vi "USO_GUI.vi"() -> ()   [LabVIEW 2014]
uses:
  gfitsio/cfitsio-bitpix.ctl
  <vilib>/Instr/_visa.llb/VISA Configure Serial Port (Instr).vi
  gfitsio/gfitsio.lvlib
  <vilib>/gmath/NI_Gmath.lvlib
panel:
  out "Start time Array":timestamp[](array[timestamp])
  out "End time Array":timestamp[](array[timestamp])
  in  "Voltage-Retardance file path for lcvr2":path
  in  "Start observation session":bool
  out "LCVR closing\nvariable":T1(array[cluster])
  out "LCVR variable":T2
  out "Current Lcvr Temp":dbl
  out "volt set of lcvr 2":dbl[](array[numeric]) format="%_6g"
  out "volt set of lcvr 1":dbl[](array[numeric]) format="%_6g"
  in  "Voltage-Retardance file path for lcvr1":path
  in  "LCVR Set Temperature":dbl=21.0 min=10.0 max=50.0
  out "Buf no 2":bool
  out "Buf no 1":bool
  out "hout":u64
  in  "OpenStructureIn":T3={"Size"=88, "InterfaceType"=1, "Camera Number"=0, "CameraNumAtInterface"=0, "OpenFlags"=[], "OpenDWFlags"=[], "OpenPtrs"=[]} {"InterfaceType" items=["IEEE1394/FireWire", "IEEE1394/FireWire", "Matrox Helios CameraLink", "SiliconSoftware MicroEnableIII CL", "National Instruments CameraLink", "Gigabit Ethernet", "USB", "SiliconSoftware MicroEnable IV CL", "Reserved", "Reserved", "Generic CameraLink with CLSER.DLL"]}
  out "Buff_no 2":i16
  out "Buff_no1":i16
  in  "Close USO software":bool
  in  "spectroscopy/spectropolarimetry tab":enum32{"Spectroscopy", "Spectropolarimetry"}(tab) caption="Tab Control"
  in  "Slide":cluster{i32, i32}(slide)={16384, 0} scale=0.0..16400.0
  in  "Display Intensity control":bool
  in  "Control Pannel":T4
  in  "Cam Exp (msec)":dbl
  out "Cam Delay (msec)":dbl
  in  "Scan distance (1=10nm)":dbl min=-6000.0 max=6000.0 step=0.01
  in  "Scan steps":dbl=190.0
  out "Steps performed":i32(slide) max=190 scale=0.0..190.0
  in  "Start Spectroscopy":bool
  in  "Stop Spectroscopy":bool
  out "CCD Display":i32[][](graph)
  out "Data is stored in the folder.........":path
  in  "accept intensity":bool
  in  "Averaging \nNum":dbl=1.0
  in  "Image averaging":enum32{"Per scan", "Per Polarisation"}(radio)
  in  "LCVR Temperature in deg C\n      Set         Current":dbl[](array[numeric]) min=0.0 max=50.0
  in  "Slide sp":cluster{i32, i32}(slide)={16384, 0} scale=0.0..16400.0
  in  "accept intensity sp":bool
  out "Data is stored in the folder sp.........":path
  out "CCD Display sp":i32[][](graph)
  in  "Stop Spectroscopy sp":bool
  in  "Start Spectroscopy sp":bool
  out "Steps performed sp":i32(slide) max=190 scale=0.0..10.0
  in  "Scan steps sp":dbl=190.0
  in  "Scan distance (1=10nm) sp":dbl min=-6000.0 max=6000.0 step=0.01
  out "Cam Delay (msec) sp":dbl
  in  "Cam Exp (msec) sp":dbl
  in  "Display Intensity control sp":bool
  in  "Control Pannel sp":T4
  out "Motor Variable":T5
  out "Cam Variable":T6
  in  "Move step size(1=10nm)":i32=100
  in  "VISA Refnum in":refnum<visa-resource-name>
  in  "DELAY (ms) in":u32=50
  in  "CONTROLLER Number":string="1"
  out "Status":string
  in  "Apply":bool
  in  "InterfaceType":u32(ring)=6 items=["Ethernet"=5, "USB"=6]
  in  "Finish":bool
  out "Cam Detail":T7
  in  "Delay in msec":u32 max=4233600000
  in  "Exposure in msec":u32=30 min=500 max=4233600000
  in  "Initialise Device":u16(ring)=3 items=["Camera", "Liquid crystal", "Scan mirror", "--FF--"]
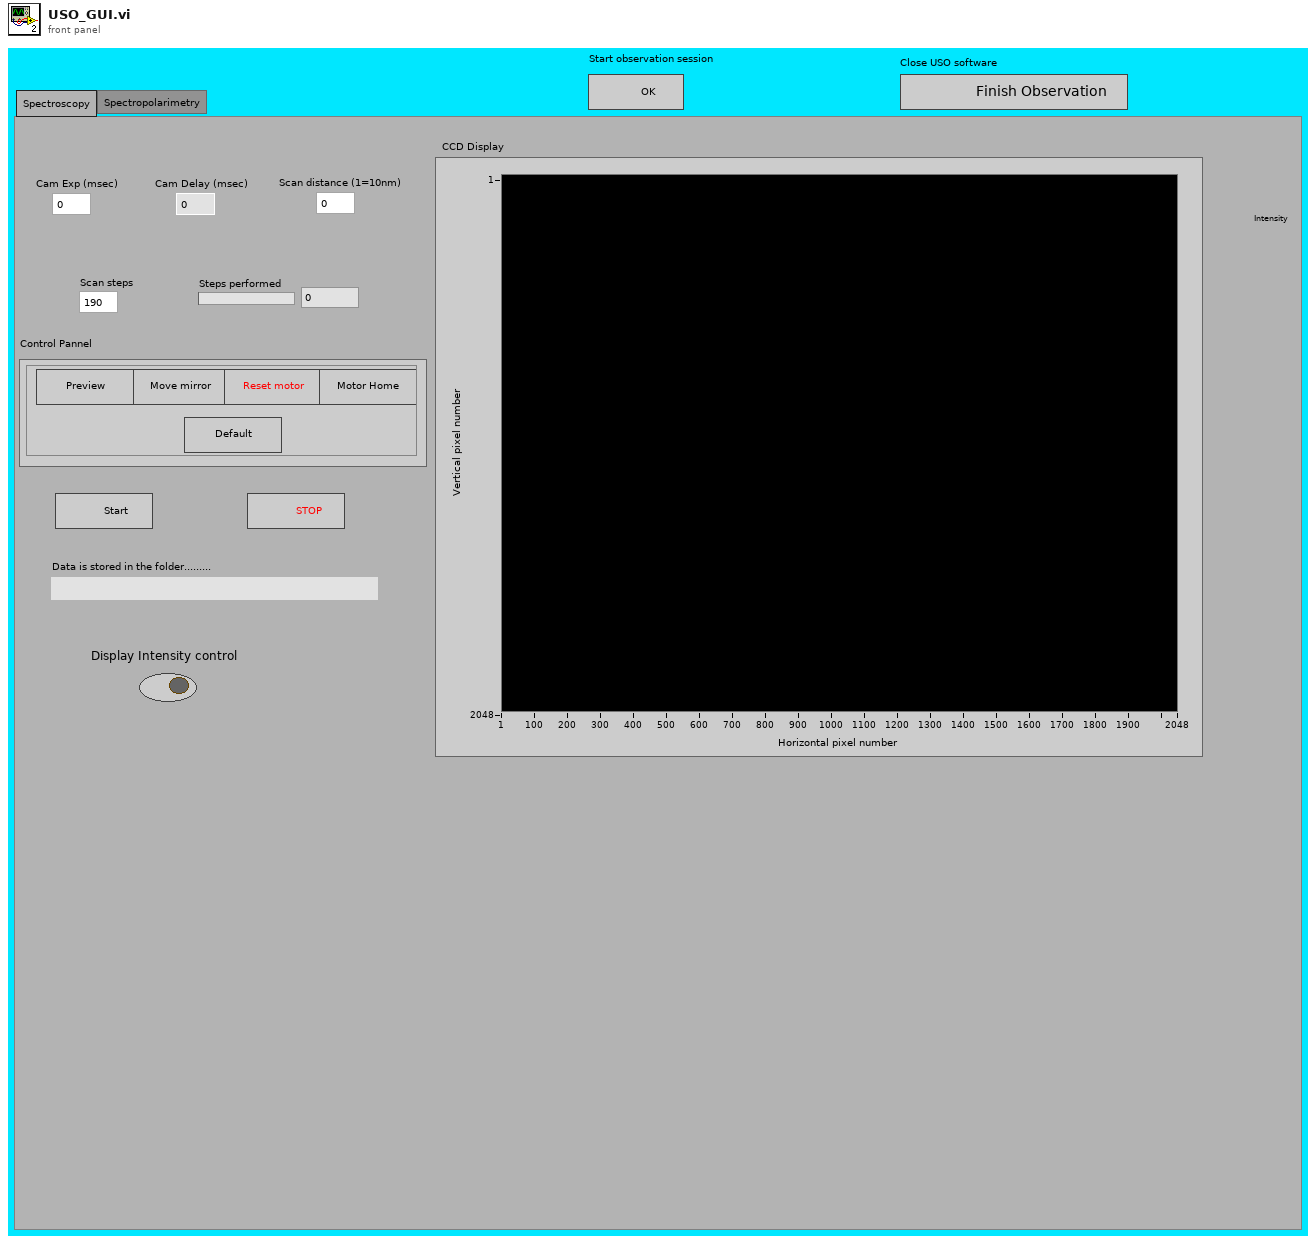
[diagram p1: front panel]
types:
  T1 = cluster{"Device Handle":u32, "Pipe 0 Handle":u32, "Pipe 1 Handle":u32}[]
  T2 = cluster{"Open USB I/O Stuff":cluster{"Device Handle":u32, "Pipe 0 Handle":u32, "Pipe 1 Handle":u32}, "volt set of lcvr 1":dbl[], "volt set of lcvr 2":dbl[], "LCVR Set Temperature":dbl, "Current Lcvr Temp":dbl}
  T3 = cluster{"Size":u16, "InterfaceType":u16, "Camera Number":u16, "CameraNumAtInterface":u16, "OpenFlags":u16[], "OpenDWFlags":u32[], "OpenPtrs":u32[]}
  T4 = cluster{"Move mirror":bool, "Preview":bool, "reset motor":bool, "motor home":bool, "Restore default values":bool}
  T5 = cluster{"Dup Controller #":string, "VISA Refnum out":refnum<visa-resource-name>, "DELAY (ms) out":u32, "Move step size":i32, "error out":errorcluster}
  T6 = cluster{"hout":u64, "ErrorOut":errorcluster, "Description":cluster{"Size":u16, "SensorTypeDESC":u16, "SensorSubtypeDESC":u16, "MaxHorizontalResStdDESC":u16, "MaxVerticalResStdDESC":u16, "MaxHorizontalResExtDESC":u16, "MaxVerticalResExtDESC":u16, "DynResDESC":u16, "MaxBinHorzDESC":u16, "BinHorzStepDESC":bool, "MaxBinVertDESC":u16, "BinVertStepDESC":bool, "ROIHorzStepDESC":u16, "ROIVertStepDESC":u16, "NumADCDESC":u16, "IRDESC":bool, "MinDelayDESC":u32, "MaxDelayDESC":u32, "MinDelayStepDESC":u32, "MinExpoDESC":u32, "MaxExpoDESC":u32, "MinExpoStepDESC":u32, "MinDelayIRDESC":u32, "MaxDelayIRDESC":u32, "MinExpoIRDESC":u32, "MaxExpoIRDESC":u32, "TimeTableDESC":bool, "DoubleImageDESC":bool, "MinCoolSetDESC":i16, "MaxCoolSetDESC":i16, "MDefaultCoolSetDESC":i16, "PowerDownModeDESC":bool, "OffsetRegDESC":bool, "ColorPattern":cluster{"UpperLeftColor":u8, "UpperRightColor":u8, "LowerLeftColor":u8, "LowerRightColor":u8}, "PatternTypeDESC":bool, "PixelRates":u32[], "CoversionFactors":u16[], "Reserved":u32[], "NoiseFilterCapable":bool, "HotPixelCapable":bool, "HotPixelWithNoiseFilter":bool, "ASCIITimeCapable":bool, "Extended Description":bool, "Get Extended":bool, "Reserved Flag 1":bool, "Reserved Flag 2":bool}}
  T7 = cluster{"Size":u16, "SensorTypeDESC":u16, "SensorSubtypeDESC":u16, "MaxHorizontalResStdDESC":u16, "MaxVerticalResStdDESC":u16, "MaxHorizontalResExtDESC":u16, "MaxVerticalResExtDESC":u16, "DynResDESC":u16, "MaxBinHorzDESC":u16, "BinHorzStepDESC":bool, "MaxBinVertDESC":u16, "BinVertStepDESC":bool, "ROIHorzStepDESC":u16, "ROIVertStepDESC":u16, "NumADCDESC":u16, "IRDESC":bool, "MinDelayDESC":u32, "MaxDelayDESC":u32, "MinDelayStepDESC":u32, "MinExpoDESC":u32, "MaxExpoDESC":u32, "MinExpoStepDESC":u32, "MinDelayIRDESC":u32, "MaxDelayIRDESC":u32, "MinExpoIRDESC":u32, "MaxExpoIRDESC":u32, "TimeTableDESC":bool, "DoubleImageDESC":bool, "MinCoolSetDESC":i16, "MaxCoolSetDESC":i16, "MDefaultCoolSetDESC":i16, "PowerDownModeDESC":bool, "OffsetRegDESC":bool, "ColorPattern":cluster{"UpperLeftColor":u8, "UpperRightColor":u8, "LowerLeftColor":u8, "LowerRightColor":u8}, "PatternTypeDESC":bool, "PixelRates":u32[], "CoversionFactors":u16[], "Reserved":u32[], "NoiseFilterCapable":bool, "HotPixelCapable":bool, "HotPixelWithNoiseFilter":bool, "ASCIITimeCapable":bool, "Extended Description":bool, "Get Extended":bool, "Reserved Flag 1":bool, "Reserved Flag 2":bool}
  T8 = enum8{"Enabled", "Disabled", "Disabled and Grayed Out"}
  T9 = enum16{"open", "open or create", "create or replace", "create", "open (read only)"}
  T10 = cluster{"Device Handle":u32, "Pipe 0 Handle":u32, "Pipe 1 Handle":u32}
  T11 = cluster{"Open USB I/O Stuff":cluster{"Device Handle":u32, "Pipe 0 Handle":u32, "Pipe 1 Handle":u32}, "yi":dbl[], "yi":dbl[], dbl, "Temp":dbl}
  T12 = cluster{"Dup Controller #":string, "VISA Refnum out":refnum<visa-resource-name>, "DELAY (ms) out":u32, "Move step size(1=10nm)":i32, "error out":errorcluster}
  T13 = cluster{"hout":u64, "error out":errorcluster, "Description":cluster{"Size":u16, "SensorTypeDESC":u16, "SensorSubtypeDESC":u16, "MaxHorizontalResStdDESC":u16, "MaxVerticalResStdDESC":u16, "MaxHorizontalResExtDESC":u16, "MaxVerticalResExtDESC":u16, "DynResDESC":u16, "MaxBinHorzDESC":u16, "BinHorzStepDESC":bool, "MaxBinVertDESC":u16, "BinVertStepDESC":bool, "ROIHorzStepDESC":u16, "ROIVertStepDESC":u16, "NumADCDESC":u16, "IRDESC":bool, "MinDelayDESC":u32, "MaxDelayDESC":u32, "MinDelayStepDESC":u32, "MinExpoDESC":u32, "MaxExpoDESC":u32, "MinExpoStepDESC":u32, "MinDelayIRDESC":u32, "MaxDelayIRDESC":u32, "MinExpoIRDESC":u32, "MaxExpoIRDESC":u32, "TimeTableDESC":bool, "DoubleImageDESC":bool, "MinCoolSetDESC":i16, "MaxCoolSetDESC":i16, "MDefaultCoolSetDESC":i16, "PowerDownModeDESC":bool, "OffsetRegDESC":bool, "ColorPattern":cluster{"UpperLeftColor":u8, "UpperRightColor":u8, "LowerLeftColor":u8, "LowerRightColor":u8}, "PatternTypeDESC":bool, "PixelRates":u32[], "CoversionFactors":u16[], "Reserved":u32[], "NoiseFilterCapable":bool, "HotPixelCapable":bool, "HotPixelWithNoiseFilter":bool, "ASCIITimeCapable":bool, "Extended Description":bool, "Get Extended":bool, "Reserved Flag 1":bool, "Reserved Flag 2":bool}}
  T14 = cluster{"Dup Controller # out":string, "VISA Refnum out":refnum<visa-resource-name>, "DELAY (ms) out":u32, "Move step size":i32, "error out":errorcluster}
  T15 = cluster{"Dup Controller #":string, "VISA Refnum out":refnum<visa-resource-name>, "Delay (ms) out ":u32, "Move step size":i32, "error out":errorcluster}
  T16 = cluster{"Dup Controller #":string, "Dup. VISA handle":refnum<visa-resource-name>, "DELAY (ms) out":u32, "Move step size":i32, "error out":errorcluster}
  T17 = typedef "gfitsio.lvlib/cfitsio-bitpix.ctl" = i32
  T18 = typedef "gfitsio.lvlib/gfitsio-refnum.ctl" = refnum<k1>
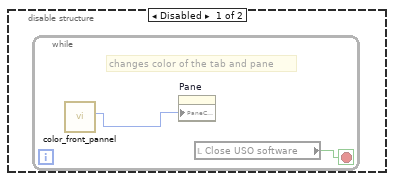
[diagram p2: hidden frame]
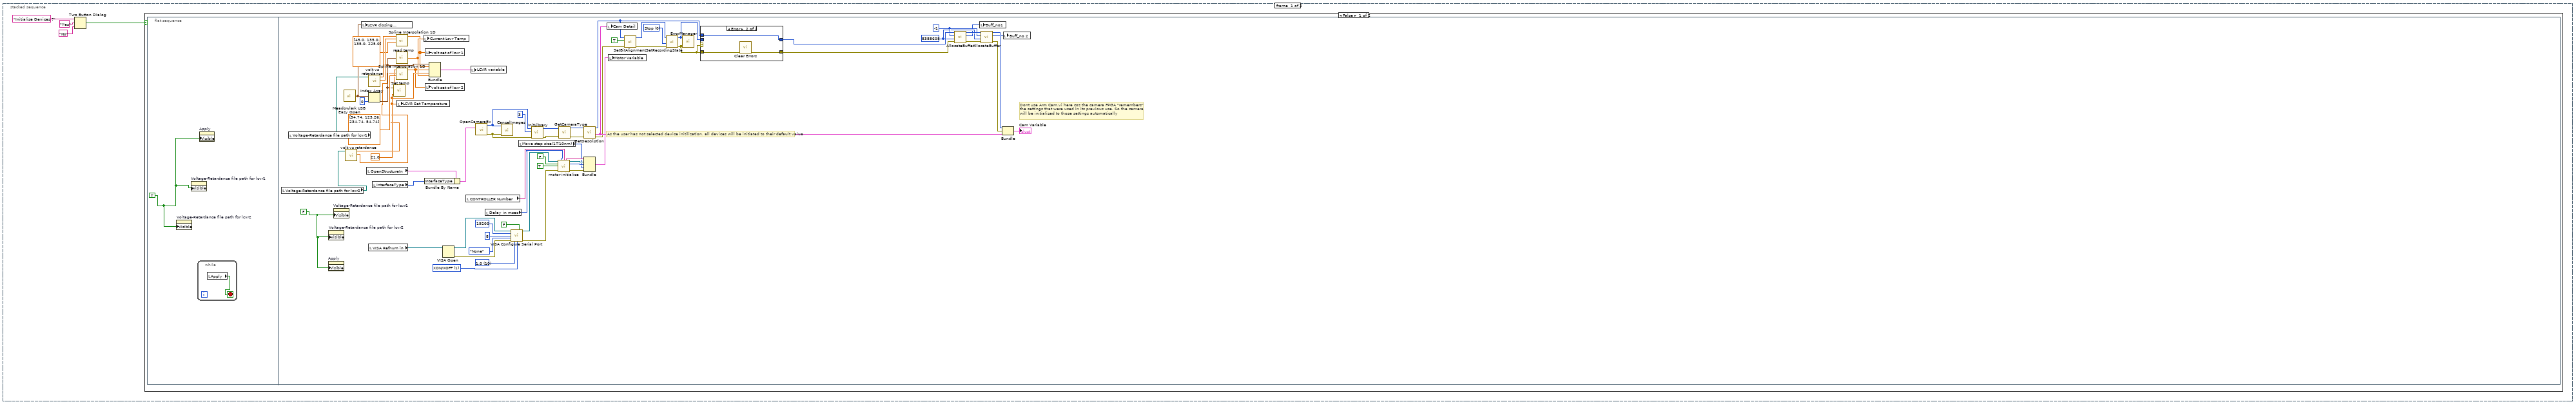
[diagram p3: hidden frame]
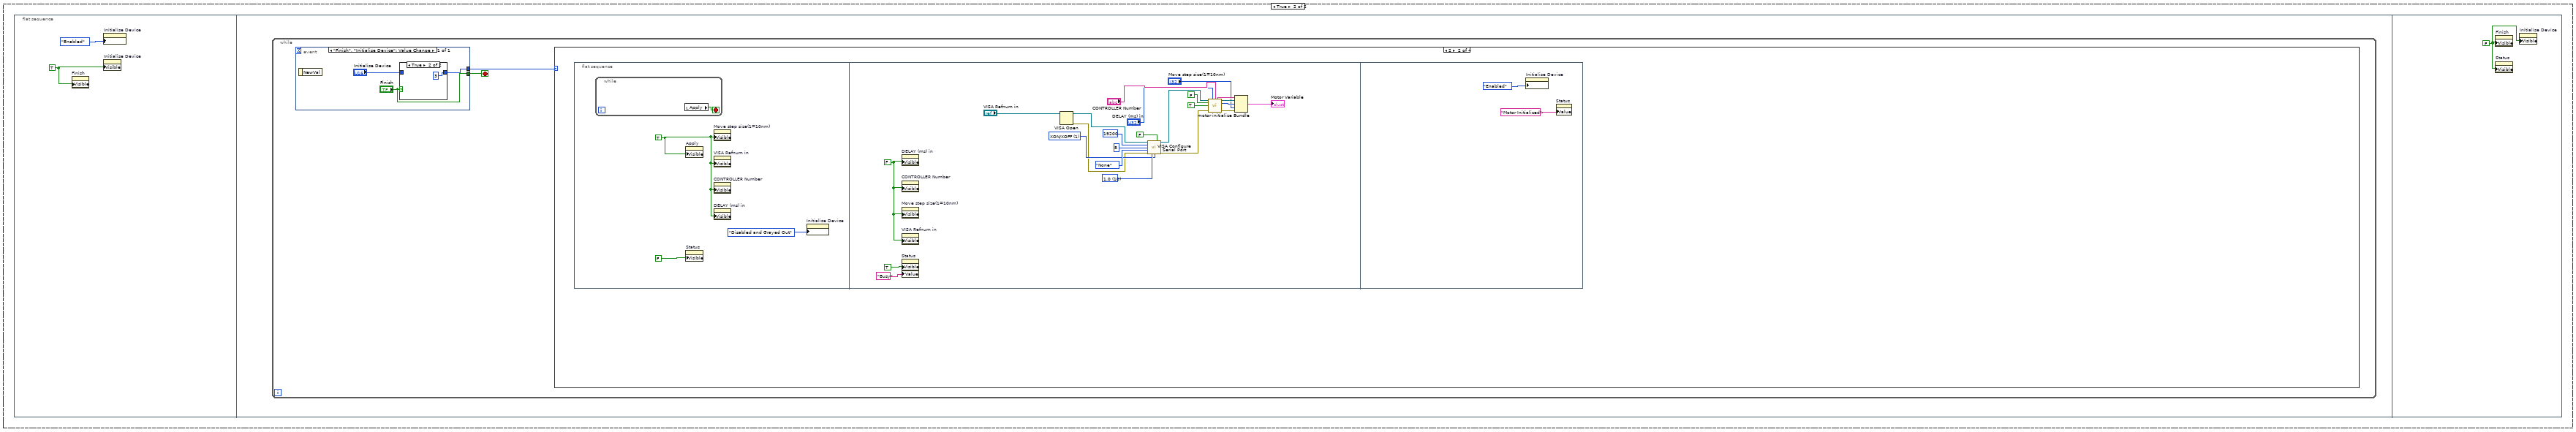
[diagram p5: hidden frame]
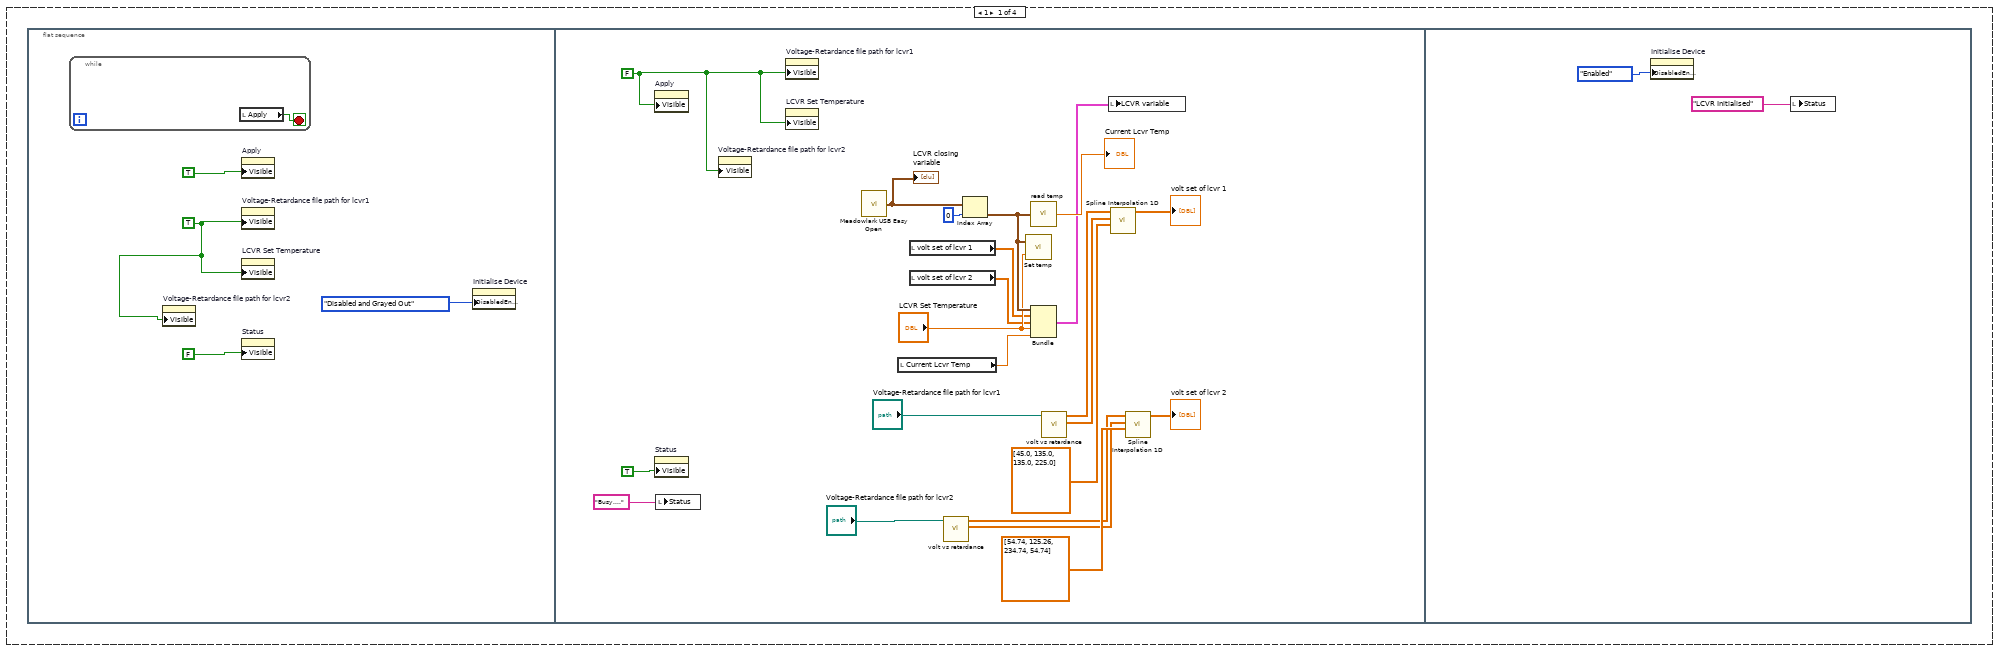
[diagram p7: hidden frame]
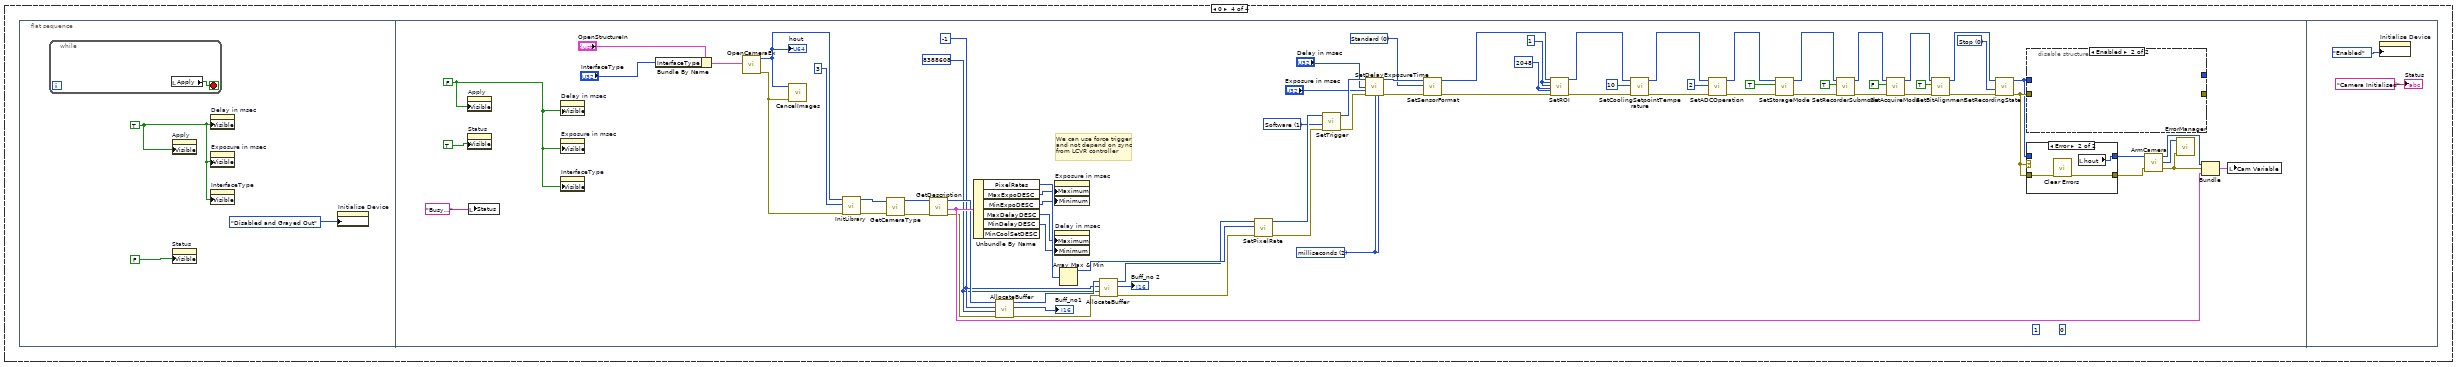
[diagram p9: hidden frame]
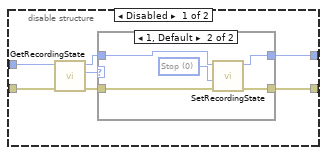
[diagram p10: hidden frame]
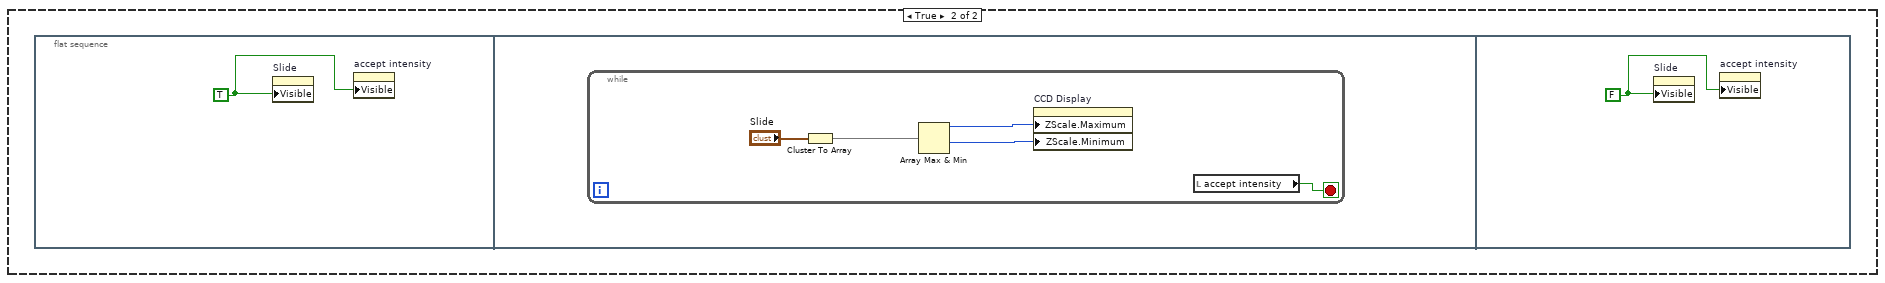
[diagram p16: hidden frame]
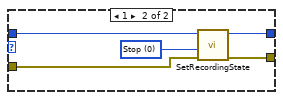
[diagram p17: hidden frame]
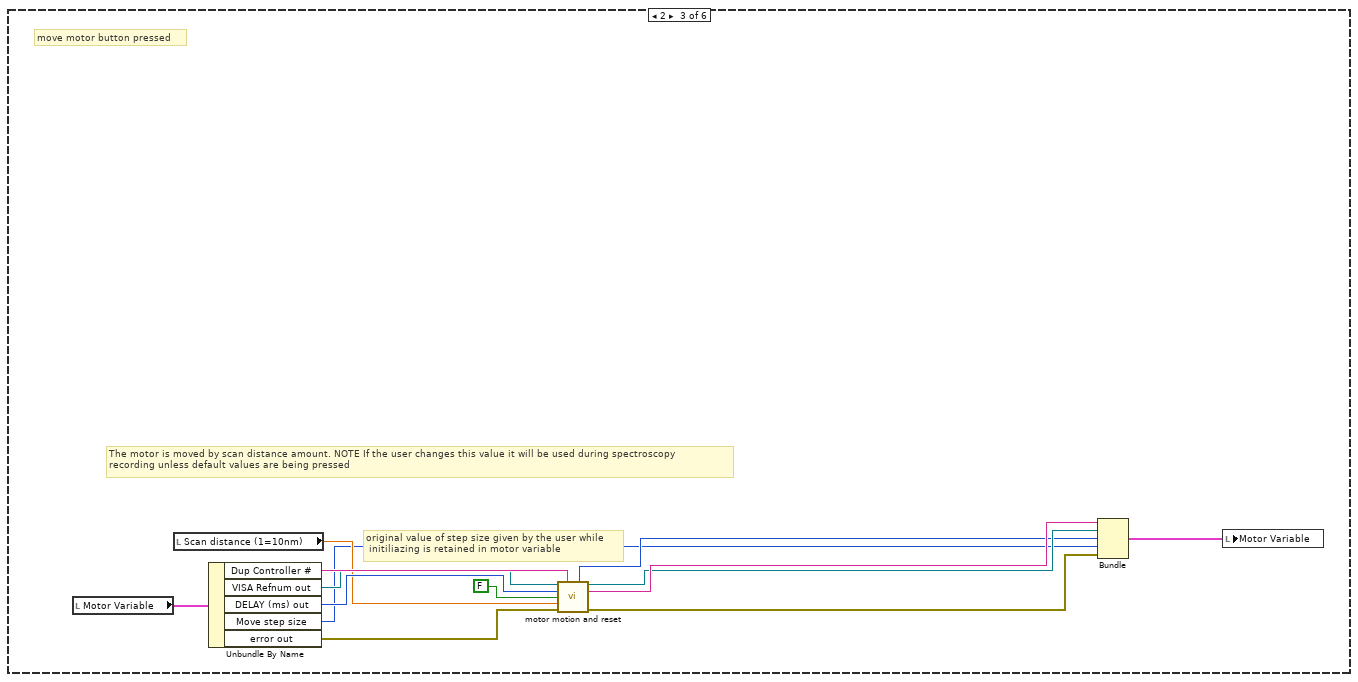
[diagram p19: hidden frame]
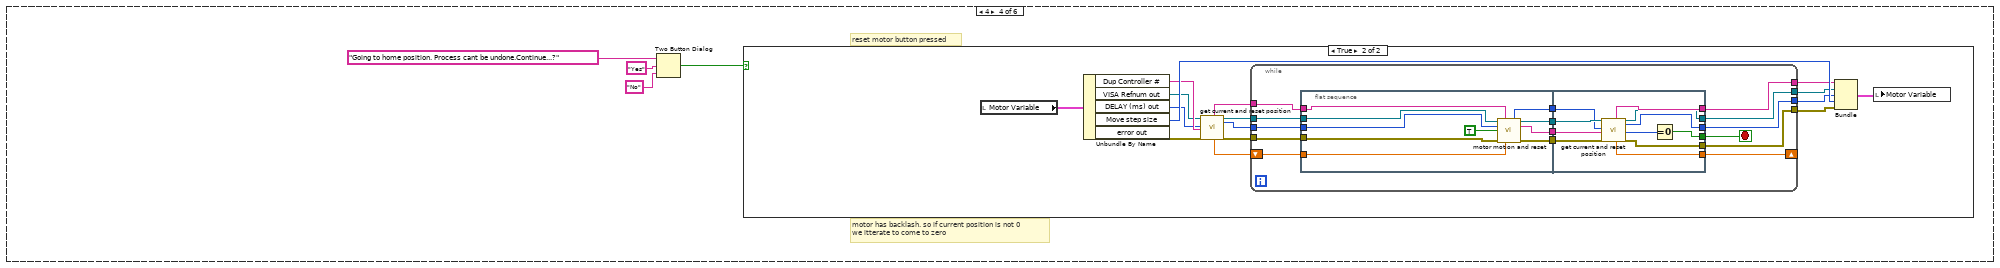
[diagram p20: hidden frame]
diagram:
  w2 = TRUE
  w3 = 2048.0 ("X Scale.Range:Maximum")
  w4 = 1.0 ("X Scale.Range:Minimum")
  w1 = FALSE
  n1 = disable-structure shown="Enabled" {
    frame Disabled {
      n2 = while {
        stop <- w6 stop-if-true
        # "changes color of the tab and pane"
        n3 = call "color_front_pannel.vi"() -> ("Resolved Color"=w5:u32)  [unwired: 11 in]
        n4 = property on="Pane" class="Pane"("PaneColor"=w5) -> ()  [unwired: 2 in, 2 out]
        n5 = local read "Close USO software"() -> (w6:bool)
      }
    }
    frame Enabled {
    }
  }
  n6 = stacked-sequence {
    frame #0 {
      n7 = Two Button Dialog(message="Initialise Devices ?", 1:"No" ("F button name (\"Cancel\")"), 2:"Yes" ("T button name (\"OK\")")) -> (T button?=w7:bool)
      n8 = case shown="False" w7 {
        frame False {
          n9 = flat-sequence {
            frame #0 {
              w11 = TRUE
              n10 = property on="Voltage-Retardance file path for lcvr2" class="Path"("Visible"=w11) -> ()  [unwired: 2 in, 2 out]
              n11 = property on="Voltage-Retardance file path for lcvr1" class="Path"("Visible"=w11) -> ()  [unwired: 2 in, 2 out]
              n12 = while {
                stop <- w12 stop-if-true
                n13 = local read "Apply"() -> (w12:bool)
              }
              n14 = property on="Apply" class="Bool (strict)"("Visible"=w11) -> ()  [unwired: 2 in, 2 out]
            }
            frame #1 {
              w13 = FALSE
              w24 = u16 1 items=["None", "XON/XOFF", "RTS/CTS", "XON/XOFF & RTS/CTS", "DTR/DSR", "XON/XOFF & DTR/DSR"] ("flow control (0:none)")
              w25 = u16 10 items=["1.0"=10, "1.5"=15, "2.0"=20] ("stop bits (10: 1 bit)")
              w39 = 21.0
              w56 = u32 8388608 ("Size")
              w57 = i16 -1 ("BufNr")
              w64 = u16 0 items=["Stop", "Run"] ("RecordingState")
              # "Dont use Arm Cam.vi here coz the camera FPGA \"remembers\"\nthe settings that were used in its previous use. So the camera \nwill be initialized to those settings automatically"
              # "As the user has not selected device initilization, all devices will be initiated to their default value"
              n15 = local read "Voltage-Retardance file path for lcvr2"() -> (w14:path)
              n16 = local read "Voltage-Retardance file path for lcvr1"() -> (w15:path)
              n17 = property on="Apply" class="Bool (strict)"("Visible"=w13) -> ()  [unwired: 2 in, 2 out]
              n18 = property on="Voltage-Retardance file path for lcvr2" class="Path"("Visible"=w13) -> ()  [unwired: 2 in, 2 out]
              n19 = property on="Voltage-Retardance file path for lcvr1" class="Path"("Visible"=w13) -> ()  [unwired: 2 in, 2 out]
              n20 = call "Meadowlark USB Easy Open.vi"() -> ("USB Device and Pipes Array"=w34:T1)  [unwired: 2 out]
              n21 = call "volt vs retardance.vi"("file path (dialog if empty)"=w14) -> ("retardance in degree(known)"=w16:dbl[], "Voltage(unknown)"=w17:dbl[])  [unwired: 9 in]
              n22 = local write "LCVR closing\nvariable"(w34) -> ()
              n23 = local read "OpenStructureIn"() -> (w51:T3)
              n24 = call "volt vs retardance.vi"("file path (dialog if empty)"=w15) -> ("retardance in degree(known)"=w44:dbl[], "Voltage(unknown)"=w43:dbl[])  [unwired: 9 in]
              n25 = Index Array(array=w34, index=0) -> (element=w40:T10)
              n26 = local read "VISA Refnum in"() -> (w20:refnum<visa-resource-name>)
              n27 = local read "InterfaceType"() -> (w49:u32)
              n28 = call "Set temp.vi"("Temp"=w39, "USB Open Device Cluster"=w40) -> ()  [unwired: 1 in]
              n29 = call <vilib>:"Spline Interpolation 1D.vi"("xi"=dbl[] [45.0, 135.0, 135.0, 225.0], "X"=w44, "Y"=w43) -> ("yi"=w37:dbl[])  [unwired: 6 in, 2 out]
              n30 = call "read temp.vi"("USB Open Device Cluster"=w40) -> ("Temp"=w38:dbl)
              n31 = call <vilib>:"Spline Interpolation 1D.vi"("xi"=dbl[] [54.74, 125.26, 234.74, 54.74], "X"=w16, "Y"=w17) -> ("yi"=w36:dbl[])  [unwired: 6 in, 2 out]
              n32 = local write "LCVR Set Temperature"(w39) -> ()
              n33 = local write "Current Lcvr Temp"(w38) -> ()
              n34 = Bundle By Name(cluster=w51, "InterfaceType"=w49) -> (w48:T3)
              n35 = local write "volt set of lcvr 1"(w37) -> ()
              n36 = local write "volt set of lcvr 2"(w36) -> ()
              n37 = Bundle("Open USB I/O Stuff"=w40, "yi"=w37, "yi"=w36, w39, "Temp"=w38) -> (w35:T11)  [unwired: 1 in]
              n38 = VISA Open(VISA resource name=w20) -> (VISA resource name=w22:refnum<visa-resource-name>, error out=w21:errorcluster)  [unwired: 4 in]
              n39 = local read "CONTROLLER Number"() -> (w71:string)
              n40 = local write "LCVR variable"(w35) -> ()
              n41 = call <userlib>:"OpenCameraEx.vi"("OpenStructureIn"=w48) -> ("error out"=w46:errorcluster, "hout"=w47:u64)  [unwired: 3 in, 2 out]
              n42 = local read "Delay in msec"() -> (w72:u32)
              n43 = call <userlib>:"CancelImages.vi"("error in (no error)"=w46, "ph"=w47) -> ()  [unwired: 1 in, 3 out]
              n44 = call-poly "VISA Configure Serial Port"("VISA resource name"=w22, "Enable Termination\nChar (T)"=FALSE ("Enable Termination\nChar (T)"), "baud rate (9600)"=u32 19200, "data bits (8)"=u16 8, "parity (0:none)"=enum16{"None", "Odd", "Even", "Mark", "Space"}."None", "error in (no error)"=w21, "stop bits (10: 1 bit)"=w25, "flow control (0:none)"=w24) -> ("VISA resource name out"=w19:refnum<visa-resource-name>, "error out"=w18:errorcluster)  [unwired: 6 in]
              n45 = local read "Move step size(1=10nm)"() -> (w66:i32)
              n46 = call <userlib>:"InitLibrary.vi"("error in (no error)"=w46, "InterfaceType"=u32 3, "ph"=w47) -> ("error out"=w79:errorcluster, "hout"=w80:u64)  [unwired: 7 in]
              n47 = call "motor initialize.vi"("VISA Refnum in"=w19, "DELAY (ms) in"=w72, "CONTROLLER"=w71, "MODE"=FALSE, "MOTOR OFF/ON"=TRUE, "error in (no error)"=w18) -> ("Dup Controller #"=w70:string, "VISA Refnum out"=w68:refnum<visa-resource-name>, "DELAY (ms) out"=w67:u32, "error out"=w65:errorcluster)  [unwired: 2 in, 4 out]
              n48 = call <userlib>:"GetCameraType.vi"("ph"=w80, "error in (no error)"=w79) -> ("hout"=w78:u64, "error out"=w77:errorcluster)  [unwired: 1 in, 2 out]
              n49 = call <userlib>:"GetDescription.vi"("ErrorIn"=w77, "ph"=w78) -> ("ErrorOut"=w30:errorcluster, "Description"=w76:T7, "hout"=w32:u64)  [unwired: 2 in, 1 out]
              n50 = Bundle("Dup Controller #"=w70, "VISA Refnum out"=w68, "DELAY (ms) out"=w67, "Move step size(1=10nm)"=w66, "error out"=w65) -> (w69:T12)  [unwired: 1 in]
              n51 = local write "Cam Detail"(w76) -> ()
              n52 = local write "Motor Variable"(w69) -> ()
              n53 = call <userlib>:"SetBitAlignment.vi"("error in (no error)"=w30, "BitAlignent"=TRUE, "ph"=w32) -> ("error out"=w29:errorcluster, "hout"=w31:u64)  [unwired: 2 in, 1 out]
              n54 = call <userlib>:"SetRecordingState.vi"("ErrorIn"=w29, "RecordingState"=w64, "ph"=w31) -> ("ErrorOut"=w52:errorcluster, "hout"=w53:u64)  [unwired: 2 in, 1 out]
              n55 = call <userlib>:"ErrorManager.vi"("ErrorIn"=w52, "ErrorCode"=w53) -> ()  [unwired: 3 in, 1 out]
              n56 = case shown="Error" w52 {
                tunnel: [w82 w84] -> w60
                tunnel: w52 -> [w82 w85]
                tunnel: w53 -> [w81 _]
                tunnel: [w81 w83] -> w63
                tunnel: w32 -> [_ w83]
                frame No Error {
                }
                frame Error {
                  n57 = call <vilib>:"Clear Errors.vi"("error in (no error)"=w85) -> ("error out"=w84:errorcluster)  [unwired: 5 in, 1 out]
                }
              }
              n58 = call <userlib>:"AllocateBuffer.vi"("error in (no error)"=w60, "Size"=w56, "BufNr"=w57, "ph"=w63) -> ("error out"=w59:errorcluster, "BufNrOut"=w55:i16, "hout"=w62:u64)  [unwired: 2 in, 3 out]
              n59 = local write "Buff_no1"(w55) -> ()
              n60 = call <userlib>:"AllocateBuffer.vi"("error in (no error)"=w59, "Size"=w56, "BufNr"=w57, "ph"=w62) -> ("error out"=w58:errorcluster, "BufNrOut"=w54:i16, "hout"=w61:u64)  [unwired: 2 in, 3 out]
              n61 = Bundle("hout"=w61, "error out"=w58, "Description"=w76) -> (→"Cam Variable":T13)  [unwired: 1 in]
              n62 = local write "Buff_no 2"(w54) -> ()
            }
          }
        }
        frame True {
          n63 = flat-sequence {
            frame #0 {
              w87 = TRUE
              n64 = property on="Finish" class="Bool"("Visible"=w87) -> ()  [unwired: 2 in, 2 out]
              n65 = property on="Initialise Device" class="Ring (strict)"("DisabledEnum"=T8."Enabled" ("Disabled")) -> ()  [unwired: 2 in, 2 out]
              n66 = property on="Initialise Device" class="Ring (strict)"("Visible"=w87) -> ()  [unwired: 2 in, 2 out]
            }
            frame #1 {
              n67 = while {
                stop <- w89 stop-if-true
                n68 = event shown="[0] \"Finish\", \"Initialise Device\": Value Change" {
                  selector: _ -> [_]
                  dyn-events: _ -> [_]
                  timeout: _ -> [_]
                  tunnel: ["Finish"] -> w89
                  tunnel: [w91] -> w88
                  event "Finish", "Initialise Device": Value Change {
                    n69 = event-data() -> ()  [unwired: 1 in, 1 out]
                    n70 = case shown="True" "Finish" {
                      tunnel: [w93 3] -> w91
                      tunnel: "Initialise Device" -> [w93 _]
                      frame False {
                      }
                      frame True {
                      }
                    }
                  }
                }
                n71 = case shown="2" w88 {
                  frame 1 {
                    n72 = flat-sequence {
                      frame #0 {
                        w95 = TRUE ("Visible")
                        n73 = while {
                          stop <- w99 stop-if-true
                          n74 = local read "Apply"() -> (w99:bool)
                        }
                        n75 = property on="Voltage-Retardance file path for lcvr2" class="Path"("Visible"=w95) -> ()  [unwired: 2 in, 2 out]
                        n76 = property on="Apply" class="Bool (strict)"("Visible"=TRUE) -> ()  [unwired: 2 in, 2 out]
                        n77 = property on="Voltage-Retardance file path for lcvr1" class="Path"("Visible"=w95) -> ()  [unwired: 2 in, 2 out]
                        n78 = property on="LCVR Set Temperature" class="DigNum (strict)"("Visible"=w95) -> ()  [unwired: 2 in, 2 out]
                        n79 = property on="Status" class="Str"("Visible"=FALSE) -> ()  [unwired: 2 in, 2 out]
                        n80 = property on="Initialise Device" class="Ring (strict)"("DisabledEnum"=T8."Disabled and Grayed Out" ("Disabled")) -> ()  [unwired: 2 in, 2 out]
                      }
                      frame #1 {
                        w100 = FALSE ("Visible")
                        n81 = property on="Apply" class="Bool (strict)"("Visible"=w100) -> ()  [unwired: 2 in, 2 out]
                        n82 = property on="Status" class="Str"("Visible"=TRUE) -> ()  [unwired: 2 in, 2 out]
                        n83 = local write "Status"("Busy...." ("Status")) -> ()
                        n84 = property on="Voltage-Retardance file path for lcvr2" class="Path"("Visible"=w100) -> ()  [unwired: 2 in, 2 out]
                        n85 = property on="Voltage-Retardance file path for lcvr1" class="Path"("Visible"=w100) -> ()  [unwired: 2 in, 2 out]
                        n86 = property on="LCVR Set Temperature" class="DigNum (strict)"("Visible"=w100) -> ()  [unwired: 2 in, 2 out]
                        n87 = call "Meadowlark USB Easy Open.vi"() -> ("USB Device and Pipes Array"=w114:T1)  [unwired: 2 out]
                        "LCVR closing\nvariable" <- w114
                        n88 = local read "Current Lcvr Temp"() -> (w105:dbl)
                        n89 = local read "volt set of lcvr 1"() -> (w107:dbl[])
                        n90 = local read "volt set of lcvr 2"() -> (w108:dbl[])
                        n91 = call "volt vs retardance.vi"("file path (dialog if empty)"="Voltage-Retardance file path for lcvr2") -> ("retardance in degree(known)"=w102:dbl[], "Voltage(unknown)"=w103:dbl[])  [unwired: 9 in]
                        n92 = Index Array(array=w114, index=0) -> (element=w110:T10)
                        n93 = call "Set temp.vi"("Temp"="LCVR Set Temperature", "USB Open Device Cluster"=w110) -> ()  [unwired: 1 in]
                        n94 = call "read temp.vi"("USB Open Device Cluster"=w110) -> ("Temp"=→"Current Lcvr Temp":dbl)
                        n95 = Bundle("Open USB I/O Stuff"=w110, "volt set of lcvr 1"=w107, "volt set of lcvr 2"=w108, "LCVR Set Temperature"="LCVR Set Temperature", "Current Lcvr Temp"=w105) -> (w104:T2)  [unwired: 1 in]
                        n96 = call "volt vs retardance.vi"("file path (dialog if empty)"="Voltage-Retardance file path for lcvr1") -> ("retardance in degree(known)"=w120:dbl[], "Voltage(unknown)"=w119:dbl[])  [unwired: 9 in]
                        n97 = local write "LCVR variable"(w104) -> ()
                        n98 = call <vilib>:"Spline Interpolation 1D.vi"("xi"=dbl[] [45.0, 135.0, 135.0, 225.0], "X"=w120, "Y"=w119) -> ("yi"=→"volt set of lcvr 1":dbl[])  [unwired: 6 in, 2 out]
                        n99 = call <vilib>:"Spline Interpolation 1D.vi"("xi"=dbl[] [54.74, 125.26, 234.74, 54.74], "X"=w102, "Y"=w103) -> ("yi"=→"volt set of lcvr 2":dbl[])  [unwired: 6 in, 2 out]
                      }
                      frame #2 {
                        n100 = property on="Initialise Device" class="Ring (strict)"("DisabledEnum"=T8."Enabled" ("Disabled")) -> ()  [unwired: 2 in, 2 out]
                        n101 = local write "Status"("LCVR Initialised" ("Status")) -> ()
                      }
                    }
                  }
                  frame 2 {
                    n102 = flat-sequence {
                      frame #0 {
                        w125 = TRUE
                        n103 = while {
                          stop <- w127 stop-if-true
                          n104 = local read "Apply"() -> (w127:bool)
                        }
                        n105 = property on="Apply" class="Bool (strict)"("Visible"=w125) -> ()  [unwired: 2 in, 2 out]
                        n106 = property on="Status" class="Str"("Visible"=FALSE) -> ()  [unwired: 2 in, 2 out]
                        n107 = property on="Move step size(1=10nm)" class="DigNum (strict)"("Visible"=w125) -> ()  [unwired: 2 in, 2 out]
                        n108 = property on="VISA Refnum in" class="VISAName"("Visible"=w125) -> ()  [unwired: 2 in, 2 out]
                        n109 = property on="CONTROLLER Number" class="Str"("Visible"=w125) -> ()  [unwired: 2 in, 2 out]
                        n110 = property on="DELAY (ms) in" class="DigNum (strict)"("Visible"=w125) -> ()  [unwired: 2 in, 2 out]
                        n111 = property on="Initialise Device" class="Ring (strict)"("DisabledEnum"=T8."Disabled and Grayed Out" ("Disabled")) -> ()  [unwired: 2 in, 2 out]
                      }
                      frame #1 {
                        w134 = u16 1 items=["None", "XON/XOFF", "RTS/CTS", "XON/XOFF & RTS/CTS", "DTR/DSR", "XON/XOFF & DTR/DSR"] ("flow control (0:none)")
                        w135 = u16 10 items=["1.0"=10, "1.5"=15, "2.0"=20] ("stop bits (10: 1 bit)")
                        w147 = FALSE
                        n112 = property on="DELAY (ms) in" class="DigNum (strict)"("Visible"=w147) -> ()  [unwired: 2 in, 2 out]
                        n113 = property on="CONTROLLER Number" class="Str"("Visible"=w147) -> ()  [unwired: 2 in, 2 out]
                        n114 = property on="Move step size(1=10nm)" class="DigNum (strict)"("Visible"=w147) -> ()  [unwired: 2 in, 2 out]
                        n115 = property on="VISA Refnum in" class="VISAName"("Visible"=w147) -> ()  [unwired: 2 in, 2 out]
                        n116 = property on="Status" class="Str"("Visible"=TRUE, "Value"="Busy") -> ()  [unwired: 2 in, 2 out]
                        n117 = VISA Open(VISA resource name="VISA Refnum in") -> (VISA resource name=w131:refnum<visa-resource-name>, error out=w130:errorcluster)  [unwired: 4 in]
                        n118 = call-poly "VISA Configure Serial Port"("VISA resource name"=w131, "Enable Termination\nChar (T)"=FALSE ("Enable Termination\nChar (T)"), "baud rate (9600)"=u32 19200, "data bits (8)"=u16 8, "parity (0:none)"=enum16{"None", "Odd", "Even", "Mark", "Space"}."None", "error in (no error)"=w130, "stop bits (10: 1 bit)"=w135, "flow control (0:none)"=w134) -> ("VISA resource name out"=w128:refnum<visa-resource-name>, "error out"=w129:errorcluster)  [unwired: 6 in]
                        n119 = call "motor initialize.vi"("VISA Refnum in"=w128, "DELAY (ms) in"="DELAY (ms) in", "CONTROLLER"="CONTROLLER Number", "MODE"=FALSE, "MOTOR OFF/ON"=TRUE, "error in (no error)"=w129) -> ("Dup Controller #"=w144:string, "VISA Refnum out"=w143:refnum<visa-resource-name>, "DELAY (ms) out"=w142:u32, "error out"=w140:errorcluster)  [unwired: 2 in, 4 out]
                        n120 = Bundle("Dup Controller #"=w144, "VISA Refnum out"=w143, "DELAY (ms) out"=w142, "Move step size(1=10nm)"="Move step size(1=10nm)", "error out"=w140) -> (→"Motor Variable":T12)  [unwired: 1 in]
                      }
                      frame #2 {
                        n121 = property on="Initialise Device" class="Ring (strict)"("DisabledEnum"=T8."Enabled" ("Disabled")) -> ()  [unwired: 2 in, 2 out]
                        n122 = property on="Status" class="Str"("Value"="Motor Initialized" ("Status")) -> ()  [unwired: 2 in, 2 out]
                      }
                    }
                  }
                  frame 3, Default {
                    # "This is do nothing Case. Can be used to add components for the future"
                  }
                  frame 0 {
                    n123 = flat-sequence {
                      frame #0 {
                        w155 = TRUE
                        n124 = while {
                          stop <- w157 stop-if-true
                          n125 = local read "Apply"() -> (w157:bool)
                        }
                        n126 = property on="Apply" class="Bool (strict)"("Visible"=w155) -> ()  [unwired: 2 in, 2 out]
                        n127 = property on="Status" class="Str"("Visible"=FALSE) -> ()  [unwired: 2 in, 2 out]
                        n128 = property on="Delay in msec" class="DigNum (strict)"("Visible"=w155) -> ()  [unwired: 2 in, 2 out]
                        n129 = property on="Exposure in msec" class="DigNum (strict)"("Visible"=w155) -> ()  [unwired: 2 in, 2 out]
                        n130 = property on="InterfaceType" class="Ring (strict)"("Visible"=w155) -> ()  [unwired: 2 in, 2 out]
                        n131 = property on="Initialise Device" class="Ring (strict)"("DisabledEnum"=T8."Disabled and Grayed Out" ("Disabled")) -> ()  [unwired: 2 in, 2 out]
                      }
                      frame #1 {
                        w173 = u16 0 items=["Stop", "Run"] ("RecordingState")
                        w190 = u32 8388608 ("Size")
                        w191 = i16 -1 ("BufNr")
                        w199 = FALSE
                        w203 = u16 2 items=["nanoseconds", "microseconds", "milliseconds"] ("DelayTimeBase")
                        (unwired) u32 0 ("element")
                        (unwired) u16 1 ("ActSeg")
                        w212 = u16 0 items=["Standard", "Extended"] ("SensorIn")
                        w215 = u16 2048 ("ROIX1")
                        w216 = u16 1 ("ROIX0")
                        w223 = u16 1 items=["Auto", "Software", "External sequence start ", "External exposure control"] ("TriggerMode")
                        # "We can use force trigger\nand not depend on sync\nfrom LCVR controller"
                        n132 = property on="Apply" class="Bool (strict)"("Visible"=w199) -> ()  [unwired: 2 in, 2 out]
                        n133 = property on="Status" class="Str"("Visible"=TRUE) -> ()  [unwired: 2 in, 2 out]
                        n134 = local write "Status"("Busy..." ("Status")) -> ()
                        n135 = property on="Delay in msec" class="DigNum (strict)"("Visible"=w199) -> ()  [unwired: 2 in, 2 out]
                        n136 = property on="Exposure in msec" class="DigNum (strict)"("Visible"=w199) -> ()  [unwired: 2 in, 2 out]
                        n137 = property on="InterfaceType" class="Ring (strict)"("Visible"=w199) -> ()  [unwired: 2 in, 2 out]
                        n138 = Bundle By Name(cluster="OpenStructureIn", "InterfaceType"="InterfaceType") -> (w181:T3)
                        n139 = call <userlib>:"OpenCameraEx.vi"("OpenStructureIn"=w181) -> ("error out"=w168:errorcluster, "hout"=w169:u64)  [unwired: 3 in, 2 out]
                        "hout" <- w169
                        n140 = call <userlib>:"CancelImages.vi"("error in (no error)"=w168, "ph"=w169) -> ()  [unwired: 1 in, 3 out]
                        n141 = call <userlib>:"InitLibrary.vi"("error in (no error)"=w168, "InterfaceType"=u32 3, "ph"=w169) -> ("error out"=w230:errorcluster, "hout"=w231:u64)  [unwired: 7 in]
                        n142 = call <userlib>:"GetCameraType.vi"("ph"=w231, "error in (no error)"=w230) -> ("hout"=w228:u64, "error out"=w229:errorcluster)  [unwired: 1 in, 2 out]
                        n143 = call <userlib>:"GetDescription.vi"("ErrorIn"=w229, "ph"=w228) -> ("ErrorOut"=w189:errorcluster, "Description"=w196:T7, "hout"=w193:u64)  [unwired: 2 in, 1 out]
                        n144 = Unbundle By Name(w196) -> ("PixelRates"=w227:u32[], "MaxExpoDESC"=w220:u32, "MinExpoDESC"=w219:u32, "MaxDelayDESC"=w218:u32, "MinDelayDESC"=w217:u32)  [unwired: 1 out]
                        n145 = call <userlib>:"AllocateBuffer.vi"("error in (no error)"=w189, "Size"=w190, "BufNr"=w191, "ph"=w193) -> ("error out"=w188:errorcluster, "BufNrOut"=→"Buff_no1":i16, "hout"=w192:u64)  [unwired: 2 in, 3 out]
                        n146 = property on="Exposure in msec" class="DigNum (strict)"("Maximum"=w220, "Minimum"=w219) -> ()  [unwired: 2 in, 2 out]
                        n147 = property on="Delay in msec" class="DigNum (strict)"("Maximum"=w218, "Minimum"=w217) -> ()  [unwired: 2 in, 2 out]
                        n148 = Array Max & Min(array=w227) -> (max value=w226:u32)  [unwired: 3 out]
                        n149 = call <userlib>:"AllocateBuffer.vi"("error in (no error)"=w188, "Size"=w190, "BufNr"=w191, "ph"=w192) -> ("error out"=w184:errorcluster, "BufNrOut"=→"Buff_no 2":i16, "hout"=w185:u64)  [unwired: 2 in, 3 out]
                        n150 = call <userlib>:"SetPixelRate.vi"("error in (no error)"=w184, "PixelRate"=w226, "ph"=w185) -> ("error out"=w225:errorcluster, "hout"=w224:u64)  [unwired: 2 in, 1 out]
                        n151 = call <userlib>:"SetTrigger.vi"("error in (no error)"=w225, "TriggerMode"=w223, "ph"=w224) -> ("error out"=w221:errorcluster, "hout"=w222:u64)  [unwired: 2 in, 1 out]
                        n152 = call <userlib>:"SetDelayExposureTime.vi"("ph"=w222, "Delay"="Delay in msec", "Exposure"="Exposure in msec", "error in (no error)"=w221, "DelayTimeBase"=w203, "ExposureTimeBase"=w203) -> ("hout"=w213:u64, "error out"=w214:errorcluster)  [unwired: 7 in, 1 out]
                        n153 = call <userlib>:"SetSensorFormat.vi"("ErrorIn"=w214, "SensorIn"=w212, "ph"=w213) -> ("ErrorOut"=w210:errorcluster, "hout"=w211:u32)  [unwired: 2 in, 1 out]
                        n154 = call <userlib>:"SetROI.vi"("ph"=w211, "ROIX0"=w216, "ROIY0"=w216, "ROIX1"=w215, "ROIY1"=w215, "error in (no error)"=w210) -> ("hout"=w208:u64, "error out"=w209:errorcluster)  [unwired: 12 in]
                        n155 = call <userlib>:"SetCoolingSetpointTemperature.vi"("error in (no error)"=w209, "CoolSet"=i16 10, "ph"=w208) -> ("error out"=w207:errorcluster, "hout"=w206:u64)  [unwired: 2 in, 1 out]
                        n156 = call <userlib>:"SetADCOperation.vi"("error in (no error)"=w207, "ADCOperation"=u16 2, "ph"=w206) -> ("error out"=w178:errorcluster, "hout"=w179:u64)  [unwired: 2 in, 1 out]
                        n157 = call <userlib>:"SetStorageMode.vi"("error in (no error)"=w178, "StorageMode"=TRUE, "ph"=w179) -> ("error out"=w165:errorcluster, "hout"=w167:u64)  [unwired: 2 in, 1 out]
                        n158 = call <userlib>:"SetRecorderSubmode.vi"("error in (no error)"=w165, "RecorderSubMode"=TRUE, "ph"=w167) -> ("error out"=w164:errorcluster, "hout"=w166:u64)  [unwired: 2 in, 1 out]
                        n159 = call <userlib>:"SetAcquireMode.vi"("error in (no error)"=w164, "UseAcquireEnable"=FALSE, "ph"=w166) -> ("error out"=w160:errorcluster, "hout"=w162:u64)  [unwired: 2 in, 1 out]
                        n160 = call <userlib>:"SetBitAlignment.vi"("error in (no error)"=w160, "BitAlignent"=TRUE, "ph"=w162) -> ("error out"=w159:errorcluster, "hout"=w161:u64)  [unwired: 2 in, 1 out]
                        n161 = call <userlib>:"SetRecordingState.vi"("ErrorIn"=w159, "RecordingState"=w173, "ph"=w161) -> ("ErrorOut"=w175:errorcluster, "hout"=w174:u64)  [unwired: 2 in, 1 out]
                        n162 = disable-structure shown="Enabled" {
                          disable-tunnel: [w235 _] -> _
                          disable-tunnel: [w234 _] -> _
                          disable-tunnel: w175 -> [w233 _]
                          disable-tunnel: w174 -> [w232 _]
                          frame Disabled {
                            n163 = call <userlib>:"GetRecordingState.vi"("ErrorIn"=w233, "ph"=w232) -> ("ErrorOut"=w238:errorcluster, "Error"=w236:i32, "hout"=w237:u64)  [unwired: 2 in, 1 out]
                            n164 = case shown="1, Default" w236 {
                              tunnel: [w240 w244] -> w235
                              tunnel: [w239 w243] -> w234
                              tunnel: w238 -> [w239 w242]
                              tunnel: w237 -> [w240 w241]
                              frame 0 {
                              }
                              frame 1, Default {
                                w245 = u16 0 items=["Stop", "Run"] ("RecordingState")
                                n165 = call <userlib>:"SetRecordingState.vi"("ErrorIn"=w242, "RecordingState"=w245, "ph"=w241) -> ("ErrorOut"=w243:errorcluster, "hout"=w244:u64)  [unwired: 2 in, 1 out]
                              }
                            }
                          }
                          frame Enabled {
                          }
                        }
                        n166 = case shown="Error" w175 {
                          tunnel: w174 -> [w246 _]
                          tunnel: [w247 w249] -> w171
                          tunnel: w175 -> [w247 w250]
                          tunnel: [w246 w248] -> w172
                          frame No Error {
                          }
                          frame Error {
                            n167 = call <vilib>:"Clear Errors.vi"("error in (no error)"=w250) -> ("error out"=w249:errorcluster)  [unwired: 5 in, 1 out]
                            n168 = local read "hout"() -> (w248:u64)
                          }
                        }
                        n169 = call <userlib>:"ArmCamera.vi"("error in (no error)"=w171, "ph"=w172) -> ("error out"=w176:errorcluster, "ErrorCode"=w177:i32, "hout"=w194:u64)  [unwired: 1 in]
                        n170 = call <userlib>:"ErrorManager.vi"("ErrorIn"=w176, "ErrorCode"=w177) -> ()  [unwired: 3 in, 1 out]
                        n171 = Bundle("hout"=w194, "error out"=w176, "Description"=w196) -> (w197:T13)  [unwired: 1 in]
                        n172 = local write "Cam Variable"(w197) -> ()
                      }
                      frame #2 {
                        n173 = property on="Initialise Device" class="Ring (strict)"("DisabledEnum"=T8."Enabled" ("Disabled")) -> ()  [unwired: 2 in, 2 out]
                        "Status" <- "Camera Initialised" ("String")
                      }
                    }
                  }
                }
              }
            }
            frame #2 {
              w253 = FALSE
              n174 = property on="Finish" class="Bool"("Visible"=w253) -> ()  [unwired: 2 in, 2 out]
              n175 = property on="Status" class="Str"("Visible"=w253) -> ()  [unwired: 2 in, 2 out]
              n176 = property on="Initialise Device" class="Ring (strict)"("Visible"=w253) -> ()  [unwired: 2 in, 2 out]
            }
          }
        }
      }
    }
    frame #1 {
      w254 = TRUE ("Visible")
      n177 = local read "Exposure in msec"() -> (w260:u32)
      n178 = local read "LCVR variable"() -> (w258:T2)
      n179 = local read "Delay in msec"() -> (w261:u32)
      n180 = property on="spectroscopy/spectropolarimetry tab" class="TabCtl (strict)"("Visible"=w254) -> ()  [unwired: 2 in, 2 out]
      n181 = property on="Close USO software" class="Bool (strict)"("Visible"=w254) -> ()  [unwired: 2 in, 2 out]
      n182 = property on="Start observation session" class="Bool (strict)"("Visible"=w254) -> ()  [unwired: 2 in, 2 out]
      n183 = property on="Cam Exp (msec)" class="DigNum (strict)"("Value"=w260) -> ()  [unwired: 2 in, 2 out]
      n184 = property on="Cam Exp (msec) sp" class="DigNum (strict)"("Value"=w260) -> ()  [unwired: 2 in, 2 out]
      n185 = property on="Cam Delay (msec) sp" class="DigNum (strict)"("Value"=w261) -> ()  [unwired: 2 in, 2 out]
      n186 = property on="Cam Delay (msec)" class="DigNum (strict)"("Value"=w261) -> ()  [unwired: 2 in, 2 out]
      n187 = local read "Move step size(1=10nm)"() -> (w259:i32)
      n188 = Unbundle By Name(w258) -> ("LCVR Set Temperature"=w257:dbl, "Current Lcvr Temp"=w256:dbl)
      n189 = while {
        stop <- w263 stop-if-true
        # "Setup greyscale palette for intensity graph display: Color = i*(0x01 + 0x100 + 0x10000)"
        n190 = while {
          tunnel: [w1530] -> w262
          stop <- w1531 stop-if-true
          n191 = local read "Start observation session"() -> (w1532:bool)
          n192 = local read "Close USO software"() -> (w1530:bool)
          n193 = Or(x=w1530, y=w1532) -> (x .or. y?=w1531:bool)
        }
        n194 = for {
          N: 256 -> [_]
          tunnel: [w1533] -> w265 mode=indexing
          i -> [w1534]
          n195 = Multiply(x=65793, y=w1534) -> (x*y=w1533:i32)
        }
        n196 = property on="CCD Display" class="IntGraph (strict)"("Color Table"=w265) -> ()  [unwired: 2 in, 2 out]
        n197 = property on="CCD Display sp" class="IntGraph (strict)"("Color Table"=w265) -> ()  [unwired: 2 in, 2 out]
        n198 = case shown="False" w262 {
          frame False {
            n199 = local read "spectroscopy/spectropolarimetry tab"() -> (w267:enum32{"Spectroscopy", "Spectropolarimetry"})
            n200 = case shown="\"Spectropolarimetry\"" w267 {
              frame "Spectroscopy", Default {
                n201 = flat-sequence {
                  tunnel: [w470] -> w274
                  tunnel: [w469] -> w273
                  tunnel: [w468] -> w272
                  tunnel: [w465] -> w271
                  tunnel: w274 -> [w493]
                  tunnel: w273 -> [w488]
                  tunnel: w272 -> [w494]
                  tunnel: w271 -> [w492]
                  tunnel: [w491] -> w270
                  tunnel: [w490] -> w269
                  tunnel: [w489] -> w268
                  tunnel: w270 -> [w601]
                  tunnel: w269 -> [w605]
                  tunnel: w268 -> [w602]
                  frame #0 {
                    n202 = while {
                      stop <- w276 stop-if-true
                      n203 = while {
                        tunnel: [w283] -> w276
                        tunnel: [w286] -> w275
                        stop <- w277 stop-if-true
                        n204 = local read "Control Pannel"() -> (w284:T4)
                        n205 = Unbundle By Name(w284) -> ("Preview"=w282:bool, "Move mirror"=w281:bool, "reset motor"=w280:bool, "motor home"=w279:bool, "Restore default values"=w278:bool)
                        n206 = local read "Start Spectroscopy"() -> (w283:bool)
                        n207 = Compound Arithmetic op=OR(w282, w281, w280, w279, w278, w283) -> (w277:bool)
                        n208 = Build Array(w282, w281, w280, w279, w278) -> (w285:bool[])
                        n209 = Boolean Array To Number(Boolean array=w285) -> (number=w286:u32)
                      }
                      n210 = case shown="1" w275 {
                        frame 0, Default {
                        }
                        frame 1 {
                          w322 = u16 2 items=["nanoseconds", "microseconds", "milliseconds"] ("DelayTimeBase")
                          w307 = u32 8388608
                          # "This gives a privew image for correction or change in exposure time. NOTE exposure time set here\nwill be taken for spectroscopy unless user presses the default values button"
                          # "Preview button pressed"
                          n211 = local read "Cam Variable"() -> (w328:T6)
                          n212 = local read "Display Intensity control"() -> (w287:bool)
                          n213 = local read "Cam Delay (msec)"() -> (w300:dbl)
                          n214 = Unbundle By Name(w328) -> ("hout"=w326:u64, "ErrorOut"=w325:errorcluster, "Description"=w323:T7)
                          n215 = property on="Cam Exp (msec)" class="DigNum (strict)"() -> ("Value"=w327:dbl)  [unwired: 2 in, 2 out]
                          n216 = case shown="False" w287 {
                            frame False {
                            }
                            frame True {
                              n217 = flat-sequence {
                                frame #0 {
                                w331 = TRUE
                                n218 = property on="Slide" class="Slide (strict)"("Visible"=w331) -> ()  [unwired: 2 in, 2 out]
                                n219 = property on="accept intensity" class="Bool (strict)"("Visible"=w331) -> ()  [unwired: 2 in, 2 out]
                                }
                                frame #1 {
                                n220 = while {
                                stop <- w332 stop-if-true
                                n221 = Cluster To Array(cluster="Slide") -> (array=w336:i32[])
                                n222 = Array Max & Min(array=w336) -> (max value=w335:i32, min value=w334:i32)  [unwired: 2 out]
                                n223 = property on="CCD Display" class="IntGraph (strict)"("ZScale.Maximum"=w335, "ZScale.Minimum"=w334) -> ()  [unwired: 2 in, 2 out]
                                n224 = local read "accept intensity"() -> (w332:bool)
                                }
                                }
                                frame #2 {
                                w337 = FALSE
                                n225 = property on="Slide" class="Slide (strict)"("Visible"=w337) -> ()  [unwired: 2 in, 2 out]
                                n226 = property on="accept intensity" class="Bool (strict)"("Visible"=w337) -> ()  [unwired: 2 in, 2 out]
                                }
                              }
                            }
                          }
                          n227 = call <userlib>:"SetDelayExposureTime.vi"("ph"=w326, "Delay"=w300, "Exposure"=w327, "error in (no error)"=w325, "DelayTimeBase"=w322, "ExposureTimeBase"=w322) -> ("hout"=w315:u64, "error out"=w314:errorcluster)  [unwired: 7 in, 1 out]
                          n228 = call <userlib>:"GetRecordingState.vi"("ErrorIn"=w314, "ph"=w315) -> ("ErrorOut"=w311:errorcluster, "RecordingState"=w313:u16, "hout"=w312:u64)  [unwired: 2 in, 1 out]
                          n229 = case shown="0, Default" w313 {
                            tunnel: w312 -> [w339 w343]
                            tunnel: w311 -> [w338 w342]
                            tunnel: [w339 w341] -> w310
                            tunnel: [w338 w340] -> w309
                            frame 0, Default {
                            }
                            frame 1 {
                              w344 = u16 0 items=["Stop", "Run"] ("RecordingState")
                              n230 = call <userlib>:"SetRecordingState.vi"("ErrorIn"=w342, "RecordingState"=w344, "ph"=w343) -> ("ErrorOut"=w340:errorcluster, "hout"=w341:u64)  [unwired: 2 in, 1 out]
                            }
                          }
                          n231 = call <userlib>:"ArmCamera.vi"("error in (no error)"=w309, "ph"=w310) -> ("error out"=w304:errorcluster, "hout"=w306:u64)  [unwired: 2 out]
                          n232 = local read "Buff_no 2"() -> (w308:i16)
                          n233 = local read "Buff_no1"() -> (w321:i16)
                          n234 = call <userlib>:"ClearRAMSegment.vi"("error in (no error)"=w304, "ph"=w306) -> ("error out"=w303:errorcluster, "hout"=w305:u64)  [unwired: 1 in, 1 out]
                          n235 = call <userlib>:"AllocateBuffer.vi"("error in (no error)"=w303, "Size"=w307, "BufNr"=w308, "ph"=w305) -> ()  [unwired: 2 in, 6 out]
                          n236 = call <userlib>:"AllocateBuffer.vi"("error in (no error)"=w303, "Size"=w307, "BufNr"=w321, "ph"=w305) -> ("error out"=w319:errorcluster, "hout"=w320:u64)  [unwired: 2 in, 4 out]
                          n237 = call <userlib>:"GetRecordingState.vi"("ErrorIn"=w319, "ph"=w320) -> ("ErrorOut"=w317:errorcluster, "RecordingState"=w316:u16, "hout"=w318:u64)  [unwired: 2 in, 1 out]
                          n238 = case shown="0, Default" w316 {
                            tunnel: [w348 w351] -> w302
                            tunnel: [w347 w350] -> w301
                            tunnel: w318 -> [w346 w351]
                            tunnel: w317 -> [w345 w350]
                            frame 0, Default {
                              w349 = u16 1 items=["Stop", "Run"] ("RecordingState")
                              n239 = call <userlib>:"SetRecordingState.vi"("ErrorIn"=w345, "RecordingState"=w349, "ph"=w346) -> ("ErrorOut"=w347:errorcluster, "hout"=w348:u64)  [unwired: 2 in, 1 out]
                            }
                            frame 1 {
                            }
                          }
                          n240 = local read "Buff_no1"() -> (w296:i16)
                          n241 = call <userlib>:"ForceTrigger.vi"("ph"=w302, "error in (no error)"=w301) -> ("hout"=w297:u64, "error out"=w294:errorcluster)  [unwired: 1 in, 2 out]
                          n242 = call "grab image_2.vi"("ErrorIn"=w294, "Image number"=u32 0, "BuffNr"=w296, "ph"=w297) -> ("output image"=w288:dbl[][], "error out"=w292:errorcluster, "hout"=w293:u64)  [unwired: 4 in, 1 out]
                          n243 = local write "CCD Display"(w288) -> ()
                          n244 = Array Max & Min(array=w288) -> (max value=w291:dbl)  [unwired: 3 out]
                          n245 = call <userlib>:"CancelImages.vi"("error in (no error)"=w292, "ph"=w293) -> ("error out"=w298:errorcluster, "hout"=w299:u64)  [unwired: 1 in, 1 out]
                          n246 = Bundle("hout"=w299, "error out"=w298, "Description"=w323) -> (w324:T13)  [unwired: 1 in]
                          n247 = Greater?(x=w291, y=u16 16384) -> (0:w289:bool)
                          n248 = local write "Cam Variable"(w324) -> ()
                          n249 = case shown="True" w289 {
                            frame False {
                            }
                            frame True {
                              n250 = One Button Dialog(message="Warning CCD pixels saturated. Reduce exposure\nor reduce intensity of light              ", button name ("OK")="OK") -> ()  [unwired: 1 out]
                            }
                          }
                        }
                        frame 2 {
                          # "original value of step size given by the user while\n initiliazing is retained in motor variable"
                          # "The motor is moved by scan distance amount. NOTE If the user changes this value it will be used during spectroscopy \nrecording unless default values are being pressed"
                          # "move motor button pressed"
                          n251 = local read "Motor Variable"() -> (w364:T5)
                          n252 = local read "Scan distance (1=10nm)"() -> (w358:dbl)
                          n253 = Unbundle By Name(w364) -> ("Dup Controller #"=w363:string, "VISA Refnum out"=w362:refnum<visa-resource-name>, "DELAY (ms) out"=w361:u32, "Move step size"=w352:i32, "error out"=w360:errorcluster)
                          n254 = call "motor motion and reset.vi"("VISA Refnum in"=w362, "Dup Controller # in"=w363, "DELAY (ms) in"=w361, "Reset"=FALSE, "Move step size"=w358, "error in (no error)"=w360) -> ("DELAY (ms) out"=w355:u32, "VISA Refnum out"=w356:refnum<visa-resource-name>, "Dup Controller # out"=w357:string, "error out"=w354:errorcluster)  [unwired: 4 in, 2 out]
                          n255 = Bundle("Dup Controller # out"=w357, "VISA Refnum out"=w356, "DELAY (ms) out"=w355, "Move step size"=w352, "error out"=w354) -> (w353:T14)  [unwired: 1 in]
                          n256 = local write "Motor Variable"(w353) -> ()
                        }
                        frame 4 {
                          # "motor has backlash. so if current position is not 0\nwe itterate to come to zero"
                          # "reset motor button pressed"
                          n257 = Two Button Dialog(message="Going to home position. Process cant be undone.Continue...?", 1:"No" ("F button name (\"Cancel\")"), 2:"Yes" ("T button name (\"OK\")")) -> (T button?=w368:bool)
                          n258 = case shown="True" w368 {
                            frame False {
                            }
                            frame True {
                              n259 = local read "Motor Variable"() -> (w384:T5)
                              n260 = Unbundle By Name(w384) -> ("Dup Controller #"=w377:string, "VISA Refnum out"=w376:refnum<visa-resource-name>, "DELAY (ms) out"=w375:u32, "Move step size"=w383:i32, "error out"=w374:errorcluster)
                              n261 = call "get current and reset position.vi"("VISA Refnum in"=w376, "DELAY (ms) in"=w375, "Dup Controller # in"=w377, "error in (no error)"=w374) -> ("Dup Controller #"=w373:string, "Reset displacement"=w369:ext, "VISA Refnum out"=w372:refnum<visa-resource-name>, "Delay (ms) out"=w371:u32, "error out"=w370:errorcluster)  [unwired: 9 in, 2 out]
                              n262 = while {
                                tunnel: [w395] -> w381
                                tunnel: [w394] -> w380
                                tunnel: [w393] -> w379
                                tunnel: [w392] -> w378
                                shift-right: [w390] -> _
                                shift-left: w369 -> [w385]
                                tunnel: w373 -> [w389]
                                tunnel: w372 -> [w388]
                                tunnel: w371 -> [w387]
                                tunnel: w370 -> [w386]
                                stop <- w391 stop-if-true
                                n263 = flat-sequence {
                                tunnel: [w408] -> w399
                                tunnel: [w407] -> w398
                                tunnel: [w406] -> w397
                                tunnel: [w405] -> w396
                                tunnel: w389 -> [w404]
                                tunnel: w388 -> [w403]
                                tunnel: w387 -> [w402]
                                tunnel: w386 -> [w401]
                                tunnel: w385 -> [w400]
                                tunnel: w399 -> [w420]
                                tunnel: w398 -> [w419]
                                tunnel: w397 -> [w417]
                                tunnel: w396 -> [w418]
                                tunnel: [w416] -> w395
                                tunnel: [w415] -> w394
                                tunnel: [w414] -> w393
                                tunnel: [w413] -> w392
                                tunnel: [w411] -> w391
                                tunnel: [w410] -> w390
                                frame #0 {
                                n264 = call "motor motion and reset.vi"("VISA Refnum in"=w403, "Dup Controller # in"=w404, "DELAY (ms) in"=w402, "Reset"=TRUE, "error in (no error)"=w401, "Reset displacement"=w400) -> ("DELAY (ms) out"=w406:u32, "VISA Refnum out"=w407:refnum<visa-resource-name>, "Dup Controller # out"=w408:string, "error out"=w405:errorcluster)  [unwired: 4 in, 2 out]
                                }
                                frame #1 {
                                n265 = call "get current and reset position.vi"("VISA Refnum in"=w419, "DELAY (ms) in"=w417, "Dup Controller # in"=w420, "error in (no error)"=w418) -> ("Dup Controller #"=w416:string, "Reset displacement"=w410:ext, "VISA Refnum out"=w414:refnum<visa-resource-name>, "Delay (ms) out"=w415:u32, "Current position"=w412:i32, "error out"=w413:errorcluster)  [unwired: 9 in, 1 out]
                                n266 = Equal To 0?(x=w412) -> (x = 0?=w411:bool)
                                }
                                }
                              }
                              n267 = Bundle("Dup Controller #"=w381, "VISA Refnum out"=w379, "Delay (ms) out"=w380, "Move step size"=w383, "error out"=w378) -> (w382:T15)  [unwired: 1 in]
                              n268 = local write "Motor Variable"(w382) -> ()
                            }
                          }
                        }
                        frame 8 {
                          # "This case makes the current position of the motor as its home."
                          # "Motor home button pressed"
                          n269 = Two Button Dialog(message="This operation cant be undone. Continue...? ", 1:"No" ("F button name (\"Cancel\")"), 2:"Yes" ("T button name (\"OK\")")) -> (T button?=w424:bool)
                          n270 = case shown="True" w424 {
                            frame False {
                            }
                            frame True {
                              n271 = local read "Motor Variable"() -> (w435:T5)
                              n272 = Unbundle By Name(w435) -> ("Dup Controller #"=w429:string, "VISA Refnum out"=w434:refnum<visa-resource-name>, "DELAY (ms) out"=w433:u32, "Move step size"=w427:i32, "error out"=w431:errorcluster)
                              n273 = call "go home.vi"("error in (no error)"=w431, "HOME"=TRUE, "DELAY (ms) in"=w433, "VISA Refnum in"=w434) -> ("error out"=w428:errorcluster, "DELAY (ms) out"=w426:u32, "Dup. VISA handle"=w430:refnum<visa-resource-name>)  [unwired: 5 in]
                              n274 = Bundle("Dup Controller #"=w429, "Dup. VISA handle"=w430, "DELAY (ms) out"=w426, "Move step size"=w427, "error out"=w428) -> (w425:T16)  [unwired: 1 in]
                              n275 = local write "Motor Variable"(w425) -> ()
                            }
                          }
                        }
                        frame 16 {
                          # "Restore default button pressed"
                          n276 = Two Button Dialog(message="Restore values feed during device initialization?. This process cant be undone. Continue...?", 1:"Make current as default" ("F button name (\"Cancel\")"), 2:"Restored default" ("T button name (\"OK\")")) -> (T button?=w436:bool)
                          n277 = case shown="False" w436 {
                            frame False {
                              n278 = local read "Cam Exp (msec)"() -> (w444:dbl)
                              n279 = local read "Scan distance (1=10nm)"() -> (w443:dbl)
                              n280 = local write "Exposure in msec"(w444) -> ()
                              n281 = local read "Motor Variable"() -> (w442:T5)
                              n282 = local write "Move step size(1=10nm)"(w443) -> ()
                              n283 = To Long Integer(number=w443) -> (32bit integer=w441:i32)
                              n284 = Bundle(cluster=w442, "Move step size"=w441) -> (w440:T5)  [unwired: 4 in]
                              n285 = local write "Motor Variable"(w440) -> ()
                            }
                            frame True {
                              w451 = u16 2 items=["nanoseconds", "microseconds", "milliseconds"] ("DelayTimeBase")
                              n286 = local read "Cam Variable"() -> (w446:T6)
                              n287 = local read "Move step size(1=10nm)"() -> (w456:i32)
                              n288 = local read "Exposure in msec"() -> (w453:u32)
                              n289 = local read "Delay in msec"() -> (w449:u32)
                              n290 = Unbundle By Name(w446) -> ("hout"=w455:u64, "ErrorOut"=w454:errorcluster)
                              n291 = property on="Scan distance (1=10nm)" class="DigNum (strict)"("Value"=w456) -> ()  [unwired: 2 in, 2 out]
                              n292 = property on="Cam Exp (msec)" class="DigNum (strict)"("Value"=w453) -> ()  [unwired: 2 in, 2 out]
                              n293 = call <userlib>:"SetDelayExposureTime.vi"("ph"=w455, "Delay"=w449, "Exposure"=w453, "error in (no error)"=w454, "DelayTimeBase"=w451) -> ("hout"=w450:u64, "error out"=w452:errorcluster)  [unwired: 8 in, 1 out]
                              n294 = call <userlib>:"ArmCamera.vi"("error in (no error)"=w452, "ph"=w450) -> ("error out"=w447:errorcluster, "hout"=w448:u64)  [unwired: 2 out]
                              n295 = Bundle(cluster=w446, "hout"=w448, "ErrorOut"=w447) -> (w445:T6)  [unwired: 1 in]
                              n296 = local write "Cam Variable"(w445) -> ()
                            }
                          }
                        }
                      }
                    }
                  }
                  frame #1 {
                    n297 = local read "Cam Variable"() -> (w472:T6)
                    n298 = Unbundle By Name(w472) -> ("hout"=w464:u64, "ErrorOut"=w463:errorcluster)
                    n299 = local read "Buff_no 2"() -> (w462:i16)
                    n300 = call <userlib>:"AllocateBuffer.vi"("error in (no error)"=w463, "Size"=u32 8388608, "BufNr"=w462, "ph"=w464) -> ("error out"=w460:errorcluster, "BufNrOut"=w470:i16, "hout"=w461:u64)  [unwired: 2 in, 3 out]
                    n301 = call <userlib>:"GetRecordingState.vi"("ErrorIn"=w460, "ph"=w461) -> ("ErrorOut"=w457:errorcluster, "RecordingState"=w459:u16, "hout"=w458:u64)  [unwired: 2 in, 1 out]
                    n302 = case shown="0, Default" w459 {
                      tunnel: [w477 w479] -> w469
                      tunnel: [w476 w478] -> w468
                      tunnel: w458 -> [w474 w479]
                      tunnel: w457 -> [w473 w478]
                      frame 0, Default {
                        w475 = u16 1 items=["Stop", "Run"] ("RecordingState")
                        n303 = call <userlib>:"SetRecordingState.vi"("ErrorIn"=w473, "RecordingState"=w475, "ph"=w474) -> ("ErrorOut"=w476:errorcluster, "hout"=w477:u64)  [unwired: 2 in, 1 out]
                      }
                      frame 1 {
                      }
                    }
                    n304 = call "File Dialog"("prompt"="Select folder in which data will be stored") -> ("selected path"=w466:path)  [unwired: 11 in, 3 out]
                    n305 = Path To String(path=w466) -> (string=w465:string)
                  }
                  frame #2 {
                    # "This section is to calculate the number of images stored in the cam ram. As FIFO is used after last image the image is stored from begining\nof the ram segment"
                    # "2"
                    # "These two loops must be saperate erlse camera ram wont be used and time\ntaken to cover field of view will become large"
                    n306 = local read "Scan steps"() -> (w487:dbl)
                    n307 = for {
                      N: w487 -> [_]
                      tunnel: w488 -> [w567]
                      shift-right: [w554] -> w490
                      shift-left: w494 -> [w566]
                      shift-right: [w558] -> w484
                      shift-left: timestamp[] [] -> [w557]
                      shift-right: [w556] -> w483
                      shift-left: timestamp[] [] -> [w555]
                      i -> [w561]
                      stop <- w565 stop-if-true
                      n308 = flat-sequence {
                        tunnel: w566 -> [w571]
                        tunnel: w567 -> [w572]
                        tunnel: [w572] -> w560
                        tunnel: [w571] -> w559
                        tunnel: [w569] -> w558
                        tunnel: w557 -> [w568]
                        tunnel: [w573] -> w564
                        tunnel: [w574] -> w563
                        tunnel: w560 -> [w576]
                        tunnel: w559 -> [w575]
                        tunnel: w564 -> [w584]
                        tunnel: w563 -> [w583]
                        tunnel: [w582] -> w554
                        tunnel: [w591] -> w556
                        tunnel: w555 -> [w590]
                        frame #0 {
                          n309 = Get Date/Time In Seconds() -> (seconds since 1Jan1904=w570:timestamp)
                          n310 = Build Array (concatenate)(w568, w570) -> (w569:timestamp[])
                        }
                        frame #1 {
                          n311 = while {
                            shift-right: [w578] -> w573
                            shift-left: w576 -> [w581]
                            shift-right: [w579] -> w574
                            shift-left: w575 -> [w580]
                            stop <- w577 continue-if-true
                            n312 = call <userlib>:"GetBusyStatus.vi"("error in (no error)"=w580, "ph"=w581) -> ("error out"=w579:errorcluster, "BusyState"=w577:bool, "hout"=w578:u64)  [unwired: 2 in, 1 out]
                          }
                        }
                        frame #2 {
                          n313 = while {
                            tunnel: w584 -> [w588]
                            shift-right: [w585] -> w582
                            shift-left: w583 -> [w586]
                            stop <- w587 stop-if-true
                            n314 = call <userlib>:"ForceTrigger.vi"("ph"=w588, "error in (no error)"=w586) -> ("Triggered"=w587:bool, "error out"=w585:errorcluster)  [unwired: 1 in, 2 out]
                          }
                        }
                        frame #3 {
                          n315 = local read "Exposure in msec"() -> (w589:u32)
                          n316 = Wait (ms)(milliseconds to wait=w589) -> ()  [unwired: 1 out]
                        }
                        frame #4 {
                          n317 = Get Date/Time In Seconds() -> (seconds since 1Jan1904=w592:timestamp)
                          n318 = Build Array (concatenate)(w590, w592) -> (w591:timestamp[])
                        }
                        frame #5 {
                          n319 = local read "Scan distance (1=10nm)"() -> (w594:dbl)
                          n320 = local read "Motor Variable"() -> (w595:T5)
                          n321 = call "helper_move_motor.vi"("Move step size"=w594, "input cluster"=w595) -> ("output cluster"=w593:T14)  [unwired: 9 in]
                          n322 = local write "Motor Variable"(w593) -> ()
                        }
                        frame #6 {
                          n323 = Wait (ms)(milliseconds to wait=u32 100) -> ()  [unwired: 1 out]
                        }
                      }
                      n324 = Increment(x=w561) -> (x+1=w562:i32)
                      n325 = local write "Steps performed"(w562) -> ()
                      n326 = local read "Stop Spectroscopy"() -> (w565:bool)
                    }
                    n327 = property on="Steps performed" class="Slide (strict)"("Scale.Maximum"=w487) -> ()  [unwired: 2 in, 2 out]
                    n328 = local write "End time Array"(w483) -> ()
                    n329 = local write "Start time Array"(w484) -> ()
                    n330 = Initialize Array(0.0 ("element"), 4 ("dimension size")) -> (w480:dbl[])
                    n331 = for {
                      N: w487 -> [w517]
                      tunnel: w488 -> [w551]
                      tunnel: w493 -> [w549]
                      tunnel: w492 -> [w548]
                      shift-right: [w542] -> w491
                      shift-left: w494 -> [w550]
                      tunnel: [w538] -> w489
                      tunnel: w480 -> [w514]
                      tunnel: w480 -> [w505]
                      i -> [w496]
                      stop <- w543 stop-if-true
                      w534 = T17 16 items=["<invalid type>"=0, "BYTE_IMG  (U8)"=8, "SHORT_IMG  (I16)"=16, "USHORT_IMG  (U16)"=20, "LONG_IMG  (I32)"=32, "ULONG_IMG  (U32)"=40, "FLOAT_IMG  (SGL)"=-32, "DOUBLE_IMG  (DBL)"=-64] ("image data type")
                      n332 = Number To Decimal String(number=w496) -> (decimal integer string=w546:string)  [unwired: 1 in]
                      n333 = call "grab image_2.vi"("ErrorIn"=w550, "Image number"=u32 0, "BuffNr"=w549, "ph"=w551) -> ("output image"=w529:dbl[][], "error out"=w542:errorcluster, "hout"=w538:u64)  [unwired: 4 in, 1 out]
                      n334 = Concatenate Strings(w548, "\\" ("string"), w546, ".fits" ("string")) -> (w544:string)
                      n335 = local write "CCD Display"(w529) -> ()
                      n336 = String To Path(string=w544) -> (path=w541:path)
                      n337 = local read "Exposure in msec"() -> (w516:u32)
                      n338 = call "gfitsio-open-create-replace-file.vi"("function (open)"=T9."open or create", "file path (dialog if empty)"=w541) -> ("error out"=w535:errorcluster, "new file path"=w528:path, "gfits refnum"=w536:T18)  [unwired: 7 in]
                      n339 = Initialize Array(i16 2048 ("element"), 2 ("dimension size")) -> (w532:i16[])
                      n340 = call "gfitsio-resize-image.vi"("image data type"=w534, "naxes"=w532, "error in (no error)"=w535, "gfits refnum"=w536) -> ("error out"=w525:errorcluster, "dup gfits refnum"=w527:T18)  [unwired: 6 in]
                      n341 = local read "End time Array"() -> (w520:timestamp[])
                      n342 = local write "Data is stored in the folder........."(w528) -> ()
                      n343 = case shown="0" w496 {
                        tunnel: [TRUE FALSE] -> w495
                        frame 0 {
                        }
                        frame 1, Default {
                        }
                      }
                      n344 = local read "Start time Array"() -> (w523:timestamp[])
                      n345 = Increment(x=w496) -> (x+1=w515:i32)
                      n346 = Index Array(array=w520, index=0) -> (element=w518:timestamp)
                      n347 = Index Array(array=w523, index=0) -> (element=w521:timestamp)
                      n348 = local read "Stop Spectroscopy"() -> (w543:bool)
                      n349 = Index Array(array=w505, index=0) -> (element=w500:dbl)
                      n350 = Index Array(array=w505, index=1) -> (element=w499:dbl)
                      n351 = Index Array(array=w505, index=2) -> (element=w498:dbl)
                      n352 = Index Array(array=w505, index=3) -> (element=w497:dbl)
                      n353 = Index Array(array=w514, index=2) -> (element=w507:dbl)
                      n354 = Index Array(array=w514, index=1) -> (element=w508:dbl)
                      n355 = Index Array(array=w514, index=3) -> (element=w506:dbl)
                      n356 = Index Array(array=w514, index=0) -> (element=w509:dbl)
                      n357 = call "fits_header.vi"("gfits refnum"=w527, "error in (no error)"=w525, "start time"=w521, "total scans"=w517, "end time"=w518, "Exposure"=w516, "lcvr1_2"=w508, "lcvr2_4"=w497, "lcvr1_4"=w506, "lcvr2_2"=w499, "lcvr1_1"=w509, "lcvr1_3"=w507, "lcvr2_1"=w500, "lcvr2_3"=w498, "Curr Scan"=w515, "Teliscope parameters"=w495) -> ("dup gfits refnum"=w526:T18, "error out"=w524:errorcluster)  [unwired: 10 in]
                      n358 = call "gfitsio-write-image-subset-i16-2d.vi"("error in (no error)"=w524, "data"=w529, "gfits refnum"=w526) -> ("error out"=w530:errorcluster, "dup gfits refnum"=w539:T18)  [unwired: 7 in]
                      n359 = call "gfitsio-close-file.vi"("error in (no error)"=w530, "gfits refnum"=w539) -> ()  [unwired: 8 in, 2 out]
                    }
                  }
                  frame #3 {
                    n360 = Merge Errors(w605, w601) -> (w604:errorcluster)
                    n361 = call <userlib>:"CancelImages.vi"("error in (no error)"=w601, "ph"=w602) -> ("error out"=w598:errorcluster, "hout"=w599:u64)  [unwired: 1 in, 1 out]
                    n362 = call <vilib>:"Simple Error Handler.vi"("error in (no error)"=w604) -> ()  [unwired: 4 in, 5 out]
                    n363 = local read "Cam Variable"() -> (w600:T6)
                    n364 = local read "Stop Spectroscopy"() -> (w603:bool)
                    n365 = Bundle(cluster=w600, "hout"=w599, "ErrorOut"=w598) -> (w597:T6)  [unwired: 1 in]
                    n366 = local write "Cam Variable"(w597) -> ()
                    n367 = case shown="False" w603 {
                      frame False {
                        n368 = Two Button Dialog(message="Spectroscopy completed successfully!!.    Reset Motor?", 1:"No" ("button name (\"OK\")"), 2:"Yes" ("T button name (\"OK\")")) -> (T button?=w606:bool)
                        n369 = case shown="True" w606 {
                          frame False {
                          }
                          frame True {
                            n370 = local read "Motor Variable"() -> (w610:T5)
                            n371 = Unbundle By Name(w610) -> ("Dup Controller #"=w620:string, "VISA Refnum out"=w619:refnum<visa-resource-name>, "DELAY (ms) out"=w618:u32, "Move step size"=w625:i32, "error out"=w617:errorcluster)
                            n372 = call "get current and reset position.vi"("VISA Refnum in"=w619, "DELAY (ms) in"=w618, "Dup Controller # in"=w620, "error in (no error)"=w617) -> ("Dup Controller #"=w616:string, "Reset displacement"=w612:ext, "VISA Refnum out"=w615:refnum<visa-resource-name>, "Delay (ms) out"=w614:u32, "error out"=w613:errorcluster)  [unwired: 9 in, 2 out]
                            n373 = while {
                              tunnel: [w636] -> w624
                              tunnel: [w635] -> w623
                              tunnel: [w634] -> w622
                              tunnel: [w633] -> w621
                              shift-right: [w631] -> _
                              shift-left: w612 -> [w626]
                              tunnel: w616 -> [w630]
                              tunnel: w615 -> [w629]
                              tunnel: w614 -> [w628]
                              tunnel: w613 -> [w627]
                              stop <- w632 stop-if-true
                              n374 = flat-sequence {
                                tunnel: [w649] -> w640
                                tunnel: [w648] -> w639
                                tunnel: [w647] -> w638
                                tunnel: [w646] -> w637
                                tunnel: w630 -> [w645]
                                tunnel: w629 -> [w644]
                                tunnel: w628 -> [w643]
                                tunnel: w627 -> [w642]
                                tunnel: w626 -> [w641]
                                tunnel: w640 -> [w661]
                                tunnel: w639 -> [w660]
                                tunnel: w638 -> [w658]
                                tunnel: w637 -> [w659]
                                tunnel: [w657] -> w636
                                tunnel: [w656] -> w635
                                tunnel: [w655] -> w634
                                tunnel: [w654] -> w633
                                tunnel: [w652] -> w632
                                tunnel: [w651] -> w631
                                frame #0 {
                                n375 = call "motor motion and reset.vi"("VISA Refnum in"=w644, "Dup Controller # in"=w645, "DELAY (ms) in"=w643, "Reset"=TRUE, "error in (no error)"=w642, "Reset displacement"=w641) -> ("DELAY (ms) out"=w647:u32, "VISA Refnum out"=w648:refnum<visa-resource-name>, "Dup Controller # out"=w649:string, "error out"=w646:errorcluster)  [unwired: 4 in, 2 out]
                                }
                                frame #1 {
                                n376 = call "get current and reset position.vi"("VISA Refnum in"=w660, "DELAY (ms) in"=w658, "Dup Controller # in"=w661, "error in (no error)"=w659) -> ("Dup Controller #"=w657:string, "Reset displacement"=w651:ext, "VISA Refnum out"=w655:refnum<visa-resource-name>, "Delay (ms) out"=w656:u32, "Current position"=w653:i32, "error out"=w654:errorcluster)  [unwired: 9 in, 1 out]
                                n377 = Equal To 0?(x=w653) -> (x = 0?=w652:bool)
                                }
                              }
                            }
                            n378 = Bundle("Dup Controller #"=w624, "VISA Refnum out"=w622, "Delay (ms) out"=w623, "Move step size"=w625, "error out"=w621) -> (w611:T15)  [unwired: 1 in]
                            n379 = local write "Motor Variable"(w611) -> ()
                          }
                        }
                      }
                      frame True {
                        n380 = local write "Stop Spectroscopy"(FALSE ("Stop Spectroscopy")) -> ()
                        n381 = Two Button Dialog(message="Spectroscopy Stopped by user. Reset motor?", 1:"No" ("F button name (\"Cancel\")"), 2:"Yes" ("T button name (\"OK\")")) -> (T button?=w663:bool)
                        n382 = case shown="False" w663 {
                          frame False {
                          }
                          frame True {
                            n383 = local read "Motor Variable"() -> (w668:T5)
                            n384 = Unbundle By Name(w668) -> ("Dup Controller #"=w677:string, "VISA Refnum out"=w676:refnum<visa-resource-name>, "DELAY (ms) out"=w675:u32, "Move step size"=w682:i32, "error out"=w674:errorcluster)
                            n385 = call "get current and reset position.vi"("VISA Refnum in"=w676, "DELAY (ms) in"=w675, "Dup Controller # in"=w677, "error in (no error)"=w674) -> ("Dup Controller #"=w673:string, "Reset displacement"=w669:ext, "VISA Refnum out"=w672:refnum<visa-resource-name>, "Delay (ms) out"=w671:u32, "error out"=w670:errorcluster)  [unwired: 9 in, 2 out]
                            n386 = while {
                              tunnel: [w693] -> w681
                              tunnel: [w692] -> w680
                              tunnel: [w691] -> w679
                              tunnel: [w690] -> w678
                              shift-right: [w688] -> _
                              shift-left: w669 -> [w683]
                              tunnel: w673 -> [w687]
                              tunnel: w672 -> [w686]
                              tunnel: w671 -> [w685]
                              tunnel: w670 -> [w684]
                              stop <- w689 stop-if-true
                              n387 = flat-sequence {
                                tunnel: [w706] -> w697
                                tunnel: [w705] -> w696
                                tunnel: [w704] -> w695
                                tunnel: [w703] -> w694
                                tunnel: w687 -> [w702]
                                tunnel: w686 -> [w701]
                                tunnel: w685 -> [w700]
                                tunnel: w684 -> [w699]
                                tunnel: w683 -> [w698]
                                tunnel: w697 -> [w718]
                                tunnel: w696 -> [w717]
                                tunnel: w695 -> [w715]
                                tunnel: w694 -> [w716]
                                tunnel: [w714] -> w693
                                tunnel: [w713] -> w692
                                tunnel: [w712] -> w691
                                tunnel: [w711] -> w690
                                tunnel: [w709] -> w689
                                tunnel: [w708] -> w688
                                frame #0 {
                                n388 = call "motor motion and reset.vi"("VISA Refnum in"=w701, "Dup Controller # in"=w702, "DELAY (ms) in"=w700, "Reset"=TRUE, "error in (no error)"=w699, "Reset displacement"=w698) -> ("DELAY (ms) out"=w704:u32, "VISA Refnum out"=w705:refnum<visa-resource-name>, "Dup Controller # out"=w706:string, "error out"=w703:errorcluster)  [unwired: 4 in, 2 out]
                                }
                                frame #1 {
                                n389 = call "get current and reset position.vi"("VISA Refnum in"=w717, "DELAY (ms) in"=w715, "Dup Controller # in"=w718, "error in (no error)"=w716) -> ("Dup Controller #"=w714:string, "Reset displacement"=w708:ext, "VISA Refnum out"=w712:refnum<visa-resource-name>, "Delay (ms) out"=w713:u32, "Current position"=w710:i32, "error out"=w711:errorcluster)  [unwired: 9 in, 1 out]
                                n390 = Equal To 0?(x=w710) -> (x = 0?=w709:bool)
                                }
                              }
                            }
                            n391 = Bundle("Dup Controller #"=w681, "VISA Refnum out"=w679, "Delay (ms) out"=w680, "Move step size"=w682, "error out"=w678) -> (w667:T15)  [unwired: 1 in]
                            n392 = local write "Motor Variable"(w667) -> ()
                          }
                        }
                      }
                    }
                  }
                }
              }
              frame "Spectropolarimetry" {
                n393 = flat-sequence {
                  tunnel: [w951] -> w731
                  tunnel: [w950] -> w730
                  tunnel: [w949] -> w729
                  tunnel: [w946] -> w728
                  tunnel: w731 -> [w971]
                  tunnel: w730 -> [w972]
                  tunnel: w729 -> [w970]
                  tunnel: w728 -> [w966]
                  tunnel: [w965] -> w727
                  tunnel: [w974] -> w726
                  tunnel: [w969] -> w725
                  tunnel: w727 -> [w1411]
                  tunnel: w726 -> [w1415]
                  tunnel: w725 -> [w1412]
                  frame #0 {
                    n394 = while {
                      stop <- w749 stop-if-true
                      n395 = while {
                        tunnel: [w760] -> w750
                        tunnel: [w751] -> w749
                        stop <- w752 stop-if-true
                        n396 = local read "Control Pannel sp"() -> (w758:T4)
                        n397 = Unbundle By Name(w758) -> ("Preview"=w757:bool, "Move mirror"=w756:bool, "reset motor"=w755:bool, "motor home"=w754:bool, "Restore default values"=w753:bool)
                        n398 = local read "Start Spectroscopy sp"() -> (w751:bool)
                        n399 = Compound Arithmetic op=OR(w757, w756, w755, w754, w753, w751) -> (w752:bool)
                        n400 = Build Array(w757, w756, w755, w754, w753) -> (w759:bool[])
                        n401 = Boolean Array To Number(Boolean array=w759) -> (number=w760:u32)
                      }
                      n402 = case shown="1" w750 {
                        frame 0, Default {
                        }
                        frame 1 {
                          w797 = u16 2 items=["nanoseconds", "microseconds", "milliseconds"] ("DelayTimeBase")
                          w782 = u32 8388608
                          # "This gives a privew image for correction or change in exposure time. NOTE exposure time set here\nwill be taken for spectroscopy unless user presses the default values button"
                          # "Preview button pressed"
                          n403 = local read "Cam Variable"() -> (w802:T6)
                          n404 = local read "Cam Delay (msec) sp"() -> (w775:dbl)
                          n405 = property on="Cam Exp (msec) sp" class="DigNum (strict)"() -> ("Value"=w761:dbl)  [unwired: 2 in, 2 out]
                          n406 = Unbundle By Name(w802) -> ("hout"=w801:u64, "ErrorOut"=w800:errorcluster, "Description"=w798:T7)
                          n407 = local read "Display Intensity control sp"() -> (w762:bool)
                          n408 = call <userlib>:"SetDelayExposureTime.vi"("ph"=w801, "Delay"=w775, "Exposure"=w761, "error in (no error)"=w800, "DelayTimeBase"=w797, "ExposureTimeBase"=w797) -> ("hout"=w790:u64, "error out"=w789:errorcluster)  [unwired: 7 in, 1 out]
                          n409 = case shown="True" w762 {
                            frame False {
                            }
                            frame True {
                              n410 = flat-sequence {
                                frame #0 {
                                w805 = TRUE
                                n411 = property on="Slide sp" class="Slide (strict)"("Visible"=w805) -> ()  [unwired: 2 in, 2 out]
                                n412 = property on="accept intensity sp" class="Bool (strict)"("Visible"=w805) -> ()  [unwired: 2 in, 2 out]
                                }
                                frame #1 {
                                n413 = while {
                                stop <- w809 stop-if-true
                                n414 = Cluster To Array(cluster="Slide sp") -> (array=w810:i32[])
                                n415 = Array Max & Min(array=w810) -> (max value=w807:i32, min value=w806:i32)  [unwired: 2 out]
                                n416 = property on="CCD Display sp" class="IntGraph (strict)"("ZScale.Maximum"=w807, "ZScale.Minimum"=w806) -> ()  [unwired: 2 in, 2 out]
                                n417 = local read "accept intensity sp"() -> (w809:bool)
                                }
                                }
                                frame #2 {
                                w811 = FALSE
                                n418 = property on="Slide sp" class="Slide (strict)"("Visible"=w811) -> ()  [unwired: 2 in, 2 out]
                                n419 = property on="accept intensity sp" class="Bool (strict)"("Visible"=w811) -> ()  [unwired: 2 in, 2 out]
                                }
                              }
                            }
                          }
                          n420 = call <userlib>:"GetRecordingState.vi"("ErrorIn"=w789, "ph"=w790) -> ("ErrorOut"=w786:errorcluster, "RecordingState"=w788:u16, "hout"=w787:u64)  [unwired: 2 in, 1 out]
                          n421 = case shown="0, Default" w788 {
                            tunnel: w787 -> [w813 w817]
                            tunnel: w786 -> [w812 w816]
                            tunnel: [w813 w815] -> w785
                            tunnel: [w812 w814] -> w784
                            frame 0, Default {
                            }
                            frame 1 {
                              w818 = u16 0 items=["Stop", "Run"] ("RecordingState")
                              n422 = call <userlib>:"SetRecordingState.vi"("ErrorIn"=w816, "RecordingState"=w818, "ph"=w817) -> ("ErrorOut"=w814:errorcluster, "hout"=w815:u64)  [unwired: 2 in, 1 out]
                            }
                          }
                          n423 = call <userlib>:"ArmCamera.vi"("error in (no error)"=w784, "ph"=w785) -> ("error out"=w779:errorcluster, "hout"=w781:u64)  [unwired: 2 out]
                          n424 = local read "Buff_no 2"() -> (w783:i16)
                          n425 = local read "Buff_no1"() -> (w796:i16)
                          n426 = call <userlib>:"ClearRAMSegment.vi"("error in (no error)"=w779, "ph"=w781) -> ("error out"=w778:errorcluster, "hout"=w780:u64)  [unwired: 1 in, 1 out]
                          n427 = call <userlib>:"AllocateBuffer.vi"("error in (no error)"=w778, "Size"=w782, "BufNr"=w783, "ph"=w780) -> ()  [unwired: 2 in, 6 out]
                          n428 = call <userlib>:"AllocateBuffer.vi"("error in (no error)"=w778, "Size"=w782, "BufNr"=w796, "ph"=w780) -> ("error out"=w794:errorcluster, "hout"=w795:u64)  [unwired: 2 in, 4 out]
                          n429 = call <userlib>:"GetRecordingState.vi"("ErrorIn"=w794, "ph"=w795) -> ("ErrorOut"=w792:errorcluster, "RecordingState"=w791:u16, "hout"=w793:u64)  [unwired: 2 in, 1 out]
                          n430 = case shown="0, Default" w791 {
                            tunnel: [w822 w825] -> w777
                            tunnel: [w821 w824] -> w776
                            tunnel: w793 -> [w820 w825]
                            tunnel: w792 -> [w819 w824]
                            frame 0, Default {
                              w823 = u16 1 items=["Stop", "Run"] ("RecordingState")
                              n431 = call <userlib>:"SetRecordingState.vi"("ErrorIn"=w819, "RecordingState"=w823, "ph"=w820) -> ("ErrorOut"=w821:errorcluster, "hout"=w822:u64)  [unwired: 2 in, 1 out]
                            }
                            frame 1 {
                            }
                          }
                          n432 = local read "Buff_no1"() -> (w771:i16)
                          n433 = call <userlib>:"ForceTrigger.vi"("ph"=w777, "error in (no error)"=w776) -> ("hout"=w772:u64, "error out"=w769:errorcluster)  [unwired: 1 in, 2 out]
                          n434 = call "grab image_2.vi"("ErrorIn"=w769, "Image number"=u32 0, "BuffNr"=w771, "ph"=w772) -> ("output image"=w763:dbl[][], "error out"=w767:errorcluster, "hout"=w768:u64)  [unwired: 4 in, 1 out]
                          n435 = Array Max & Min(array=w763) -> (max value=w766:dbl)  [unwired: 3 out]
                          n436 = local write "CCD Display sp"(w763) -> ()
                          n437 = call <userlib>:"CancelImages.vi"("error in (no error)"=w767, "ph"=w768) -> ("error out"=w773:errorcluster, "hout"=w774:u64)  [unwired: 1 in, 1 out]
                          n438 = Bundle("hout"=w774, "error out"=w773, "Description"=w798) -> (w799:T13)  [unwired: 1 in]
                          n439 = Greater?(x=w766, y=u16 16384) -> (0:w764:bool)
                          n440 = local write "Cam Variable"(w799) -> ()
                          n441 = case shown="False" w764 {
                            frame False {
                            }
                            frame True {
                              n442 = One Button Dialog(message="Warning CCD pixels saturated. Reduce exposure\nor reduce intensity of light              ", button name ("OK")="OK") -> ()  [unwired: 1 out]
                            }
                          }
                        }
                        frame 2 {
                          # "original value of step size given by the user while\n initiliazing is retained in motor variable"
                          # "The motor is moved by scan distance amount. NOTE If the user changes this value it will be used during spectroscopy \nrecording unless default values are being pressed"
                          # "move motor button pressed"
                          n443 = local read "Motor Variable"() -> (w838:T5)
                          n444 = local read "Scan distance (1=10nm) sp"() -> (w832:dbl)
                          n445 = Unbundle By Name(w838) -> ("Dup Controller #"=w837:string, "VISA Refnum out"=w836:refnum<visa-resource-name>, "DELAY (ms) out"=w835:u32, "Move step size"=w826:i32, "error out"=w834:errorcluster)
                          n446 = call "motor motion and reset.vi"("VISA Refnum in"=w836, "Dup Controller # in"=w837, "DELAY (ms) in"=w835, "Reset"=FALSE, "Move step size"=w832, "error in (no error)"=w834) -> ("DELAY (ms) out"=w829:u32, "VISA Refnum out"=w830:refnum<visa-resource-name>, "Dup Controller # out"=w831:string, "error out"=w828:errorcluster)  [unwired: 4 in, 2 out]
                          n447 = Bundle("Dup Controller # out"=w831, "VISA Refnum out"=w830, "DELAY (ms) out"=w829, "Move step size"=w826, "error out"=w828) -> (w827:T14)  [unwired: 1 in]
                          n448 = local write "Motor Variable"(w827) -> ()
                        }
                        frame 4 {
                          # "motor has backlash. so if current position is not 0\nwe itterate to come to zero"
                          # "reset motor button pressed"
                          n449 = Two Button Dialog(message="Going to home position. Process cant be undone.Continue...?", 1:"No" ("F button name (\"Cancel\")"), 2:"Yes" ("T button name (\"OK\")")) -> (T button?=w842:bool)
                          n450 = case shown="False" w842 {
                            frame False {
                            }
                            frame True {
                              n451 = local read "Motor Variable"() -> (w858:T5)
                              n452 = Unbundle By Name(w858) -> ("Dup Controller #"=w851:string, "VISA Refnum out"=w850:refnum<visa-resource-name>, "DELAY (ms) out"=w849:u32, "Move step size"=w857:i32, "error out"=w848:errorcluster)
                              n453 = call "get current and reset position.vi"("VISA Refnum in"=w850, "DELAY (ms) in"=w849, "Dup Controller # in"=w851, "error in (no error)"=w848) -> ("Dup Controller #"=w847:string, "Reset displacement"=w843:ext, "VISA Refnum out"=w846:refnum<visa-resource-name>, "Delay (ms) out"=w845:u32, "error out"=w844:errorcluster)  [unwired: 9 in, 2 out]
                              n454 = while {
                                tunnel: [w869] -> w855
                                tunnel: [w868] -> w854
                                tunnel: [w867] -> w853
                                tunnel: [w866] -> w852
                                shift-right: [w864] -> _
                                shift-left: w843 -> [w859]
                                tunnel: w847 -> [w863]
                                tunnel: w846 -> [w862]
                                tunnel: w845 -> [w861]
                                tunnel: w844 -> [w860]
                                stop <- w865 stop-if-true
                                n455 = flat-sequence {
                                tunnel: [w882] -> w873
                                tunnel: [w881] -> w872
                                tunnel: [w880] -> w871
                                tunnel: [w879] -> w870
                                tunnel: w863 -> [w878]
                                tunnel: w862 -> [w877]
                                tunnel: w861 -> [w876]
                                tunnel: w860 -> [w875]
                                tunnel: w859 -> [w874]
                                tunnel: w873 -> [w894]
                                tunnel: w872 -> [w893]
                                tunnel: w871 -> [w891]
                                tunnel: w870 -> [w892]
                                tunnel: [w890] -> w869
                                tunnel: [w889] -> w868
                                tunnel: [w888] -> w867
                                tunnel: [w887] -> w866
                                tunnel: [w885] -> w865
                                tunnel: [w884] -> w864
                                frame #0 {
                                n456 = call "motor motion and reset.vi"("VISA Refnum in"=w877, "Dup Controller # in"=w878, "DELAY (ms) in"=w876, "Reset"=TRUE, "error in (no error)"=w875, "Reset displacement"=w874) -> ("DELAY (ms) out"=w880:u32, "VISA Refnum out"=w881:refnum<visa-resource-name>, "Dup Controller # out"=w882:string, "error out"=w879:errorcluster)  [unwired: 4 in, 2 out]
                                }
                                frame #1 {
                                n457 = call "get current and reset position.vi"("VISA Refnum in"=w893, "DELAY (ms) in"=w891, "Dup Controller # in"=w894, "error in (no error)"=w892) -> ("Dup Controller #"=w890:string, "Reset displacement"=w884:ext, "VISA Refnum out"=w888:refnum<visa-resource-name>, "Delay (ms) out"=w889:u32, "Current position"=w886:i32, "error out"=w887:errorcluster)  [unwired: 9 in, 1 out]
                                n458 = Equal To 0?(x=w886) -> (x = 0?=w885:bool)
                                }
                                }
                              }
                              n459 = Bundle("Dup Controller #"=w855, "VISA Refnum out"=w853, "Delay (ms) out"=w854, "Move step size"=w857, "error out"=w852) -> (w856:T15)  [unwired: 1 in]
                              n460 = local write "Motor Variable"(w856) -> ()
                            }
                          }
                        }
                        frame 8 {
                          # "This case makes the current position of the motor as its home."
                          # "Motor home button pressed"
                          n461 = Two Button Dialog(message="This operation cant be undone. Continue...? ", 1:"No" ("F button name (\"Cancel\")"), 2:"Yes" ("T button name (\"OK\")")) -> (T button?=w898:bool)
                          n462 = case shown="True" w898 {
                            frame False {
                            }
                            frame True {
                              n463 = local read "Motor Variable"() -> (w909:T5)
                              n464 = Unbundle By Name(w909) -> ("Dup Controller #"=w903:string, "VISA Refnum out"=w908:refnum<visa-resource-name>, "DELAY (ms) out"=w907:u32, "Move step size"=w901:i32, "error out"=w905:errorcluster)
                              n465 = call "go home.vi"("error in (no error)"=w905, "HOME"=TRUE, "DELAY (ms) in"=w907, "VISA Refnum in"=w908) -> ("error out"=w902:errorcluster, "DELAY (ms) out"=w900:u32, "Dup. VISA handle"=w904:refnum<visa-resource-name>)  [unwired: 5 in]
                              n466 = Bundle("Dup Controller #"=w903, "Dup. VISA handle"=w904, "DELAY (ms) out"=w900, "Move step size"=w901, "error out"=w902) -> (w899:T16)  [unwired: 1 in]
                              n467 = local write "Motor Variable"(w899) -> ()
                            }
                          }
                        }
                        frame 16 {
                          # "Restore default button pressed"
                          n468 = Two Button Dialog(message="Restore values feed during device initialization?. This process cant be undone. Continue...?", 1:"Make current as default" ("F button name (\"Cancel\")"), 2:"Restored default" ("T button name (\"OK\")")) -> (T button?=w910:bool)
                          n469 = case shown="True" w910 {
                            frame False {
                              n470 = local read "Cam Exp (msec) sp"() -> (w918:dbl)
                              n471 = local read "Scan distance (1=10nm) sp"() -> (w917:dbl)
                              n472 = local write "Exposure in msec"(w918) -> ()
                              n473 = local read "Motor Variable"() -> (w916:T5)
                              n474 = local write "Move step size(1=10nm)"(w917) -> ()
                              n475 = To Long Integer(number=w917) -> (32bit integer=w915:i32)
                              n476 = Bundle(cluster=w916, "Move step size"=w915) -> (w914:T5)  [unwired: 4 in]
                              n477 = local write "Motor Variable"(w914) -> ()
                            }
                            frame True {
                              w926 = u16 2 items=["nanoseconds", "microseconds", "milliseconds"] ("DelayTimeBase")
                              n478 = local read "Cam Variable"() -> (w921:T6)
                              n479 = local read "Move step size(1=10nm)"() -> (w919:i32)
                              n480 = local read "Exposure in msec"() -> (w928:u32)
                              n481 = local read "Delay in msec"() -> (w924:u32)
                              n482 = Unbundle By Name(w921) -> ("hout"=w930:u64, "ErrorOut"=w929:errorcluster)
                              n483 = property on="Scan distance (1=10nm) sp" class="DigNum (strict)"("Value"=w919) -> ()  [unwired: 2 in, 2 out]
                              n484 = call <userlib>:"SetDelayExposureTime.vi"("ph"=w930, "Delay"=w924, "Exposure"=w928, "error in (no error)"=w929, "DelayTimeBase"=w926) -> ("hout"=w925:u64, "error out"=w927:errorcluster)  [unwired: 8 in, 1 out]
                              n485 = call <userlib>:"ArmCamera.vi"("error in (no error)"=w927, "ph"=w925) -> ("error out"=w922:errorcluster, "hout"=w923:u64)  [unwired: 2 out]
                              n486 = Bundle(cluster=w921, "hout"=w923, "ErrorOut"=w922) -> (w920:T6)  [unwired: 1 in]
                              n487 = local write "Cam Variable"(w920) -> ()
                            }
                          }
                        }
                      }
                    }
                  }
                  frame #1 {
                    n488 = local read "LCVR variable"() -> (w935:T2)
                    n489 = Unbundle By Name(w935) -> ("LCVR Set Temperature"=w934:dbl, "Current Lcvr Temp"=w933:dbl)
                    n490 = call "= to within Tolerance"("Operand 2"=w933, "Operand 1"=w934) -> ("Result"=w932:dynamicdata)  [unwired: 8 in, 1 out]
                    n491 = call "Convert from Dynamic Data"("Dynamic Data Type"=w932) -> ("Scalar"=w931:bool)  [unwired: 3 in]
                    n492 = case shown="False" w931 {
                      frame False {
                        n493 = One Button Dialog(message="Warning the lcvr temp \nis not equal to the set temp", button name ("OK")="OK") -> ()  [unwired: 1 out]
                      }
                      frame True {
                      }
                    }
                  }
                  frame #2 {
                    n494 = local read "Cam Variable"() -> (w953:T6)
                    n495 = local read "Buff_no 2"() -> (w943:i16)
                    n496 = Unbundle By Name(w953) -> ("hout"=w945:u64, "ErrorOut"=w944:errorcluster)
                    n497 = call <userlib>:"AllocateBuffer.vi"("error in (no error)"=w944, "Size"=u32 8388608, "BufNr"=w943, "ph"=w945) -> ("error out"=w941:errorcluster, "BufNrOut"=w951:i16, "hout"=w942:u64)  [unwired: 2 in, 3 out]
                    n498 = call <userlib>:"GetRecordingState.vi"("ErrorIn"=w941, "ph"=w942) -> ("ErrorOut"=w938:errorcluster, "RecordingState"=w940:u16, "hout"=w939:u64)  [unwired: 2 in, 1 out]
                    n499 = case shown="0, Default" w940 {
                      tunnel: [w958 w960] -> w950
                      tunnel: [w957 w959] -> w949
                      tunnel: w939 -> [w955 w960]
                      tunnel: w938 -> [w954 w959]
                      frame 0, Default {
                        w956 = u16 1 items=["Stop", "Run"] ("RecordingState")
                        n500 = call <userlib>:"SetRecordingState.vi"("ErrorIn"=w954, "RecordingState"=w956, "ph"=w955) -> ("ErrorOut"=w957:errorcluster, "hout"=w958:u64)  [unwired: 2 in, 1 out]
                      }
                      frame 1 {
                      }
                    }
                    n501 = call "File Dialog2"("prompt"="Select folder in which data will be stored") -> ("selected path"=w947:path)  [unwired: 11 in, 3 out]
                    n502 = Path To String(path=w947) -> (string=w946:string)
                  }
                  frame #3 {
                    # "This section is to calculate the number of images stored in the cam ram. As FIFO is used after last image the image is stored from begining\nof the ram segment"
                    n503 = local read "Image averaging"() -> (w973:enum32{"Per scan", "Per Polarisation"})
                    n504 = local read "Averaging \nNum"() -> (w968:dbl)
                    n505 = local read "Scan steps sp"() -> (w967:dbl)
                    n506 = property on="Steps performed sp" class="Slide (strict)"("Scale.Maximum"=w967) -> ()  [unwired: 2 in, 2 out]
                    n507 = case shown="\"Per scan\", Default" w973 {
                      tunnel: w972 -> [w985 w1142]
                      tunnel: w971 -> [w984 w1141]
                      tunnel: w970 -> [w983 w1140]
                      tunnel: [w982 w1139] -> w969
                      tunnel: w968 -> [w980 w1138]
                      tunnel: w967 -> [w981 w1137]
                      tunnel: w966 -> [w979 w1136]
                      tunnel: [w978 w1135] -> w965
                      frame "Per scan", Default {
                        n508 = local read "LCVR variable"() -> (w977:T2)
                        n509 = Unbundle By Name(w977) -> ("volt set of lcvr 1"=w976:dbl[], "volt set of lcvr 2"=w975:dbl[])
                        n510 = for {
                          N: w981 -> [w1004]
                          tunnel: w984 -> [w1055]
                          tunnel: w983 -> [w1054]
                          tunnel: w980 -> [w1002]
                          shift-right: [w1053] -> w982
                          shift-left: w985 -> [w1056]
                          tunnel: w980 -> [w1048]
                          tunnel: w979 -> [w1046]
                          tunnel: [w1028] -> w978
                          tunnel: w976 -> [w987]
                          tunnel: w975 -> [w986]
                          i -> [w989]
                          stop <- w1026 stop-if-true
                          w991 = 3 ("index")
                          w993 = 2 ("index")
                          w995 = 1 ("index")
                          w997 = 0 ("index")
                          w1024 = 2048 ("dimension size")
                          w1034 = 2048.0 ("element")
                          w1036 = T17 16 items=["<invalid type>"=0, "BYTE_IMG  (U8)"=8, "SHORT_IMG  (I16)"=16, "USHORT_IMG  (U16)"=20, "LONG_IMG  (I32)"=32, "ULONG_IMG  (U32)"=40, "FLOAT_IMG  (SGL)"=-32, "DOUBLE_IMG  (DBL)"=-64] ("image data type")
                          # "only the 1st fits file will have teliscope parameters"
                          n511 = Initialize Array(0.0 ("element"), w1024, w1024) -> (w1023:dbl[][])
                          n512 = for {
                            N: w1002 -> [_]
                            tunnel: w1055 -> [w1089]
                            shift-right: [w1084] -> w1053
                            shift-left: w1056 -> [w1090]
                            shift-right: [w1080] -> w1029
                            shift-left: w1054 -> [w1088]
                            shift-right: [w1075] -> w1052
                            shift-left: w1023 -> [w1071]
                            shift-right: [w1074] -> w1051
                            shift-left: w1023 -> [w1070]
                            shift-right: [w1073] -> w1050
                            shift-left: w1023 -> [w1069]
                            shift-right: [w1072] -> w1049
                            shift-left: w1023 -> [w1068]
                            n513 = flat-sequence {
                              tunnel: w1090 -> [w1100]
                              tunnel: w1089 -> [w1095]
                              tunnel: w1088 -> [w1099]
                              tunnel: [w1097] -> w1087
                              tunnel: [w1096] -> w1083
                              tunnel: [w1095] -> w1079
                              tunnel: [w1095] -> w1077
                              tunnel: [w1093] -> w1075
                              tunnel: w1071 -> [w1094]
                              tunnel: w1087 -> [w1111]
                              tunnel: [w1110] -> w1086
                              tunnel: w1083 -> [w1109]
                              tunnel: [w1108] -> w1082
                              tunnel: w1079 -> [w1107]
                              tunnel: [w1106] -> w1078
                              tunnel: w1077 -> [w1106]
                              tunnel: [w1103] -> w1074
                              tunnel: w1070 -> [w1104]
                              tunnel: w1086 -> [w1121]
                              tunnel: [w1120] -> w1085
                              tunnel: w1082 -> [w1119]
                              tunnel: [w1118] -> w1081
                              tunnel: w1078 -> [w1117]
                              tunnel: [w1117] -> w1076
                              tunnel: [w1114] -> w1073
                              tunnel: w1069 -> [w1115]
                              tunnel: w1085 -> [w1131]
                              tunnel: [w1130] -> w1084
                              tunnel: w1081 -> [w1129]
                              tunnel: [w1128] -> w1080
                              tunnel: w1076 -> [w1127]
                              tunnel: [w1124] -> w1072
                              tunnel: w1068 -> [w1125]
                              frame #0 {
                                n514 = call "grab image_2.vi"("ErrorIn"=w1099, "Image number"=u32 0, "BuffNr"=w1095, "ph"=w1100) -> ("output image"=w1092:dbl[][], "error out"=w1096:errorcluster, "hout"=w1097:u64)  [unwired: 4 in, 1 out]
                                n515 = To Extended Precision Float(1:w1092) -> (0:w1091:ext[][])
                                n516 = Add(x=w1091, y=w1094) -> (x+y=w1093:ext[][])
                              }
                              frame #1 {
                                n517 = call "grab image_2.vi"("ErrorIn"=w1109, "Image number"=u32 0, "BuffNr"=w1107, "ph"=w1111) -> ("output image"=w1102:dbl[][], "error out"=w1108:errorcluster, "hout"=w1110:u64)  [unwired: 4 in, 1 out]
                                n518 = To Extended Precision Float(1:w1102) -> (0:w1101:ext[][])
                                n519 = Add(x=w1101, y=w1104) -> (x+y=w1103:ext[][])
                              }
                              frame #2 {
                                n520 = call "grab image_2.vi"("ErrorIn"=w1119, "Image number"=u32 0, "BuffNr"=w1117, "ph"=w1121) -> ("output image"=w1113:dbl[][], "error out"=w1118:errorcluster, "hout"=w1120:u64)  [unwired: 4 in, 1 out]
                                n521 = To Extended Precision Float(1:w1113) -> (0:w1112:ext[][])
                                n522 = Add(x=w1112, y=w1115) -> (x+y=w1114:ext[][])
                              }
                              frame #3 {
                                n523 = call "grab image_2.vi"("ErrorIn"=w1129, "Image number"=u32 0, "BuffNr"=w1127, "ph"=w1131) -> ("output image"=w1123:dbl[][], "error out"=w1128:errorcluster, "hout"=w1130:u64)  [unwired: 4 in, 1 out]
                                n524 = To Extended Precision Float(1:w1123) -> (0:w1122:ext[][])
                                n525 = Add(x=w1122, y=w1125) -> (x+y=w1124:ext[][])
                              }
                            }
                          }
                          n526 = Number To Decimal String(number=w989) -> (decimal integer string=w1044:string)  [unwired: 1 in]
                          n527 = Concatenate Strings(w1046, "\\" ("string"), w1044, ".fits" ("string")) -> (w1042:string)
                          n528 = String To Path(string=w1042) -> (path=w1041:path)
                          n529 = Divide(x=w1051, y=w1048) -> (x/y=w1020:ext[][])
                          n530 = Divide(x=w1050, y=w1048) -> (x/y=w1018:ext[][])
                          n531 = Divide(x=w1049, y=w1048) -> (x/y=w1016:ext[][])
                          n532 = Divide(x=w1052, y=w1048) -> (x/y=w1022:ext[][])
                          n533 = To Word Integer(number=w1020) -> (16bit integer=w1019:i16[][])
                          n534 = To Word Integer(number=w1018) -> (16bit integer=w1017:i16[][])
                          n535 = To Word Integer(number=w1016) -> (16bit integer=w1015:i16[][])
                          n536 = To Word Integer(number=w1022) -> (16bit integer=w1021:i16[][])
                          n537 = local write "CCD Display sp"(w1022) -> ()
                          n538 = local read "Exposure in msec"() -> (w1009:u32)
                          n539 = local read "End time Array"() -> (w1006:timestamp[])
                          n540 = Build Array(4.0 ("element"), w1034, w1034) -> (w1033:dbl[])
                          n541 = call "gfitsio-open-create-replace-file.vi"("advisory dialog? (display:T)"=FALSE, "function (open)"=T9."open or create", "file path (dialog if empty)"=w1041) -> ("error out"=w1038:errorcluster, "gfits refnum"=w1037:T18)  [unwired: 6 in, 1 out]
                          n542 = local read "Start time Array"() -> (w1008:timestamp[])
                          n543 = Build Array(w1021, w1019, w1017, w1015) -> (w1014:i16[][][])
                          n544 = Increment(x=w989) -> (x+1=w1003:i32)
                          n545 = call "gfitsio-resize-image.vi"("image data type"=w1036, "naxes"=w1033, "error in (no error)"=w1038, "gfits refnum"=w1037) -> ("error out"=w1011:errorcluster, "dup gfits refnum"=w1013:T18)  [unwired: 6 in]
                          n546 = Index Array(array=w1006, index=w1003) -> (element=w1005:timestamp)
                          n547 = Index Array(array=w1008, index=w1003) -> (element=w1007:timestamp)
                          n548 = case shown="1, Default" w989 {
                            tunnel: [TRUE FALSE] -> w988
                            frame 0 {
                            }
                            frame 1, Default {
                            }
                          }
                          n549 = Index Array(array=w986, index=w997) -> (element=w996:dbl)
                          n550 = Index Array(array=w986, index=w991) -> (element=w990:dbl)
                          n551 = Index Array(array=w986, index=w995) -> (element=w994:dbl)
                          n552 = Index Array(array=w986, index=w993) -> (element=w992:dbl)
                          n553 = Index Array(array=w987, index=w993) -> (element=w999:dbl)
                          n554 = Index Array(array=w987, index=w995) -> (element=w1000:dbl)
                          n555 = Index Array(array=w987, index=w997) -> (element=w1001:dbl)
                          n556 = Index Array(array=w987, index=w991) -> (element=w998:dbl)
                          n557 = call "fits_header.vi"("gfits refnum"=w1013, "error in (no error)"=w1011, "start time"=w1007, "total scans"=w1004, "end time"=w1005, "Exposure"=w1009, "num of img added"=w1002, "lcvr1_2"=w1000, "lcvr2_4"=w990, "lcvr1_4"=w998, "lcvr2_2"=w994, "lcvr1_1"=w1001, "lcvr1_3"=w999, "lcvr2_1"=w996, "lcvr2_3"=w992, "Curr Scan"=w1003, "Teliscope parameters"=w988) -> ("dup gfits refnum"=w1012:T18, "error out"=w1010:errorcluster)  [unwired: 9 in]
                          n558 = for {
                            N: 4 -> [_]
                            tunnel: w1014 -> [w1065] mode=indexing
                            shift-right: [w1064] -> w1032
                            shift-left: w1012 -> [w1067]
                            shift-right: [w1063] -> w1031
                            shift-left: w1010 -> [w1066]
                            i -> [w1062]
                            w1059 = 1.0 ("element")
                            n559 = Increment(x=w1062) -> (x+1=w1060:i32)
                            n560 = Build Array(w1060, w1059, w1059) -> (w1061:dbl[])
                            n561 = call "gfitsio-write-image-subset-i16-2d.vi"("fpixel"=w1061, "error in (no error)"=w1066, "data"=w1065, "gfits refnum"=w1067) -> ("error out"=w1063:errorcluster, "dup gfits refnum"=w1064:T18)  [unwired: 6 in]
                          }
                          n562 = call "gfitsio-close-file.vi"("error in (no error)"=w1031, "gfits refnum"=w1032) -> ("error out"=w1030:errorcluster, "Path"=w1027:path)  [unwired: 8 in]
                          n563 = Merge Errors(w1030, w1029) -> (w1028:errorcluster)
                          n564 = local write "Data is stored in the folder sp........."(w1027) -> ()
                          n565 = local read "Stop Spectroscopy sp"() -> (w1026:bool)
                        }
                      }
                      frame "Per Polarisation" {
                        n566 = local read "LCVR variable"() -> (w1134:T2)
                        n567 = Unbundle By Name(w1134) -> ("volt set of lcvr 1"=w1133:dbl[], "volt set of lcvr 2"=w1132:dbl[])
                        n568 = for {
                          N: w1137 -> [w1166]
                          tunnel: w1141 -> [w1203]
                          tunnel: w1140 -> [w1202]
                          shift-right: [w1201] -> w1139
                          shift-left: w1142 -> [w1204]
                          tunnel: w1138 -> [w1165]
                          tunnel: w1136 -> [w1186]
                          tunnel: [w1178] -> w1135
                          tunnel: w1133 -> [w1144]
                          tunnel: w1132 -> [w1143]
                          i -> [w1146]
                          stop <- w1177 stop-if-true
                          w1187 = 2048.0 ("element")
                          w1189 = T17 16 items=["<invalid type>"=0, "BYTE_IMG  (U8)"=8, "SHORT_IMG  (I16)"=16, "USHORT_IMG  (U16)"=20, "LONG_IMG  (I32)"=32, "ULONG_IMG  (U32)"=40, "FLOAT_IMG  (SGL)"=-32, "DOUBLE_IMG  (DBL)"=-64] ("image data type")
                          n569 = Number To Decimal String(number=w1146) -> (decimal integer string=w1197:string)  [unwired: 1 in]
                          n570 = for {
                            N: 4 -> [_]
                            tunnel: w1204 -> [w1226]
                            tunnel: w1203 -> [w1225]
                            shift-right: [w1223] -> w1179
                            shift-left: w1202 -> [w1224]
                            tunnel: [w1222] -> w1201
                            tunnel: w1165 -> [w1217]
                            tunnel: [w1216] -> w1184 mode=indexing
                            tunnel: [w1216] -> w1175
                            w1220 = 2048 ("dimension size")
                            n571 = Initialize Array(0.0 ("element"), w1220, w1220) -> (w1219:dbl[][])
                            n572 = for {
                              N: w1217 -> [_]
                              tunnel: w1226 -> [w1236]
                              tunnel: w1225 -> [w1235]
                              shift-right: [w1232] -> w1223
                              shift-left: w1224 -> [w1233]
                              shift-right: [w1229] -> w1218
                              shift-left: w1219 -> [w1227]
                              tunnel: [w1228] -> w1222
                              n573 = call "grab image_2.vi"("ErrorIn"=w1233, "Image number"=u32 0, "BuffNr"=w1235, "ph"=w1236) -> ("output image"=w1230:dbl[][], "error out"=w1232:errorcluster, "hout"=w1228:u64)  [unwired: 4 in, 1 out]
                              n574 = To Extended Precision Float(1:w1230) -> (0:w1231:ext[][])
                              n575 = Add(x=w1227, y=w1231) -> (x+y=w1229:ext[][])
                            }
                            n576 = Divide(x=w1218, y=w1217) -> (x/y=w1216:ext[][])
                          }
                          n577 = Concatenate Strings(w1186, "\\" ("string"), w1197, ".fits" ("string")) -> (w1195:string)
                          n578 = String To Path(string=w1195) -> (path=w1194:path)
                          n579 = Build Array(4.0 ("element"), w1187, w1187) -> (w1185:dbl[])
                          n580 = call "gfitsio-open-create-replace-file.vi"("advisory dialog? (display:T)"=FALSE, "function (open)"=T9."open or create", "file path (dialog if empty)"=w1194) -> ("error out"=w1191:errorcluster, "gfits refnum"=w1190:T18)  [unwired: 6 in, 1 out]
                          n581 = local read "End time Array"() -> (w1168:timestamp[])
                          n582 = local read "Start time Array"() -> (w1170:timestamp[])
                          n583 = Increment(x=w1146) -> (x+1=w1163:i32)
                          n584 = local read "Exposure in msec"() -> (w1164:u32)
                          n585 = local write "CCD Display sp"(w1175) -> ()
                          n586 = call "gfitsio-resize-image.vi"("image data type"=w1189, "naxes"=w1185, "error in (no error)"=w1191, "gfits refnum"=w1190) -> ("error out"=w1172:errorcluster, "dup gfits refnum"=w1174:T18)  [unwired: 6 in]
                          n587 = To Word Integer(number=w1184) -> (16bit integer=w1183:i16[][][])
                          n588 = Index Array(array=w1170, index=w1163) -> (element=w1169:timestamp)
                          n589 = Index Array(array=w1168, index=w1163) -> (element=w1167:timestamp)
                          n590 = case shown="0" w1146 {
                            tunnel: [TRUE FALSE] -> w1145
                            frame 0 {
                            }
                            frame 1, Default {
                            }
                          }
                          n591 = Index Array(array=w1143, index=0) -> (element=w1153:dbl)
                          n592 = Index Array(array=w1144, index=2) -> (element=w1157:dbl)
                          n593 = Index Array(array=w1143, index=1) -> (element=w1151:dbl)
                          n594 = Index Array(array=w1144, index=1) -> (element=w1159:dbl)
                          n595 = Index Array(array=w1144, index=0) -> (element=w1161:dbl)
                          n596 = Index Array(array=w1144, index=3) -> (element=w1155:dbl)
                          n597 = Index Array(array=w1143, index=2) -> (element=w1149:dbl)
                          n598 = Index Array(array=w1143, index=3) -> (element=w1147:dbl)
                          n599 = call "fits_header.vi"("gfits refnum"=w1174, "error in (no error)"=w1172, "start time"=w1169, "total scans"=w1166, "end time"=w1167, "Exposure"=w1164, "num of img added"=w1165, "lcvr1_2"=w1159, "lcvr2_4"=w1147, "lcvr1_4"=w1155, "lcvr2_2"=w1151, "lcvr1_1"=w1161, "lcvr1_3"=w1157, "lcvr2_1"=w1153, "lcvr2_3"=w1149, "Curr Scan"=w1163, "Teliscope parameters"=w1145) -> ("dup gfits refnum"=w1173:T18, "error out"=w1171:errorcluster)  [unwired: 9 in]
                          n600 = for {
                            N: 4 -> [_]
                            tunnel: w1183 -> [w1215] mode=indexing
                            shift-right: [w1213] -> w1182
                            shift-left: w1173 -> [w1214]
                            shift-right: [w1211] -> w1181
                            shift-left: w1171 -> [w1212]
                            i -> [w1210]
                            w1208 = 1 ("element")
                            n601 = Increment(x=w1210) -> (x+1=w1209:i32)
                            n602 = Build Array(w1209, w1208, w1208) -> (w1207:i32[])
                            n603 = call "gfitsio-write-image-subset-i16-2d.vi"("fpixel"=w1207, "error in (no error)"=w1212, "data"=w1215, "gfits refnum"=w1214) -> ("error out"=w1211:errorcluster, "dup gfits refnum"=w1213:T18)  [unwired: 6 in]
                          }
                          n604 = call "gfitsio-close-file.vi"("error in (no error)"=w1181, "gfits refnum"=w1182) -> ("error out"=w1180:errorcluster, "Path"=w1176:path)  [unwired: 8 in]
                          n605 = Merge Errors(w1180, w1179) -> (w1178:errorcluster)
                          n606 = local write "Data is stored in the folder sp........."(w1176) -> ()
                          n607 = local read "Stop Spectroscopy sp"() -> (w1177:bool)
                        }
                      }
                    }
                    n608 = for {
                      N: w967 -> [_]
                      tunnel: w972 -> [w1254]
                      shift-right: [w1251] -> w974
                      shift-left: w970 -> [w1253]
                      shift-right: [w1240] -> w962
                      shift-left: timestamp[] [] -> [w1239]
                      shift-right: [w1238] -> w963
                      shift-left: timestamp[] [] -> [w1237]
                      i -> [w1244]
                      stop <- w1252 stop-if-true
                      n609 = Increment(x=w1244) -> (x+1=w1250:i32)
                      n610 = flat-sequence {
                        tunnel: "Averaging \nNum" -> [w1258]
                        tunnel: w1254 -> [w1259]
                        tunnel: w1253 -> [w1260]
                        tunnel: [w1260] -> w1243
                        tunnel: [w1259] -> w1242
                        tunnel: [w1258] -> w1241
                        tunnel: [w1256] -> w1240
                        tunnel: w1239 -> [w1255]
                        tunnel: [w1270] -> w1251
                        tunnel: w1243 -> [w1268]
                        tunnel: w1242 -> [w1269]
                        tunnel: w1241 -> [w1267]
                        tunnel: [w1399] -> w1238
                        tunnel: w1237 -> [w1398]
                        tunnel: w1249 -> [w1404]
                        tunnel: w1248 -> [w1403]
                        tunnel: [w1402] -> w1247
                        tunnel: w1246 -> [w1401]
                        frame #0 {
                          n611 = Get Date/Time In Seconds() -> (seconds since 1Jan1904=w1257:timestamp)
                          n612 = Build Array (concatenate)(w1255, w1257) -> (w1256:timestamp[])
                        }
                        frame #1 {
                          n613 = local read "LCVR variable"() -> (w1265:T2)
                          n614 = Unbundle By Name(w1265) -> ("Open USB I/O Stuff"=w1261:T10, "volt set of lcvr 1"=w1264:dbl[], "volt set of lcvr 2"=w1263:dbl[])
                          n615 = call "version.vi"("USB Open Device Cluster"=w1261) -> ("Version"=w1262:dbl)  [unwired: 10 in]
                          n616 = case shown="\"Per Polarisation\"" "Image averaging" {
                            tunnel: [w1275 w1340] -> w1270
                            tunnel: w1269 -> [w1277 w1339]
                            tunnel: w1268 -> [w1276 w1338]
                            tunnel: w1267 -> [w1278 w1337]
                            tunnel: w1261 -> [w1274 w1335]
                            tunnel: w1264 -> [w1273 w1334]
                            tunnel: w1263 -> [w1272 w1333]
                            tunnel: w1262 -> [w1271 w1332]
                            frame "Per scan", Default {
                              n617 = for {
                                N: w1278 -> [_]
                                tunnel: w1277 -> [w1286]
                                tunnel: w1276 -> [w1285]
                                tunnel: [w1284] -> w1275
                                tunnel: w1274 -> [w1283]
                                tunnel: w1273 -> [w1282]
                                tunnel: w1272 -> [w1281]
                                tunnel: w1271 -> [w1279]
                                stop <- w1280 stop-if-true
                                n618 = for {
                                N: 4 -> [_]
                                tunnel: w1286 -> [w1295]
                                tunnel: w1285 -> [w1294]
                                tunnel: [w1293] -> w1284
                                tunnel: w1283 -> [w1292]
                                tunnel: w1282 -> [w1291]
                                tunnel: w1281 -> [w1290]
                                tunnel: w1279 -> [w1289]
                                i -> [w1296]
                                n619 = flat-sequence {
                                tunnel: w1289 -> [w1300]
                                tunnel: w1290 -> [w1304]
                                tunnel: w1291 -> [w1305]
                                tunnel: w1292 -> [w1303]
                                tunnel: w1296 -> [w1307]
                                tunnel: w1296 -> [w1306]
                                tunnel: w1295 -> [w1318]
                                tunnel: w1294 -> [w1317]
                                tunnel: [w1316] -> w1288
                                tunnel: [w1330] -> w1293
                                tunnel: w1288 -> [w1330]
                                frame #0 {
                                # "simultaneous change in volt in two channels is not possible thus a frame sequence is put"
                                # "I found that this setteling time is nessary for proper polarimetry"
                                n620 = Index Array(array=w1305, index=w1306) -> (element=w1297:dbl)
                                n621 = Index Array(array=w1304, index=w1307) -> (element=w1301:dbl)
                                n622 = flat-sequence {
                                tunnel: [w1314] -> w1298
                                tunnel: w1297 -> [w1311]
                                tunnel: w1300 -> [w1313]
                                tunnel: 1 ("LC Channel") -> [w1312]
                                tunnel: w1297 -> [_]
                                tunnel: w1303 -> [w1314]
                                tunnel: w1300 -> [w1310]
                                tunnel: 2 ("LC Channel") -> [w1309]
                                tunnel: w1301 -> [w1308]
                                tunnel: w1298 -> [_]
                                frame #0 {
                                n623 = call <userlib>:"Meadowlark USB Set Voltage.VI"("LC Voltage"=w1308, "LC Channel"=w1309, "FW Version"=w1310, "USB Open Device Cluster"=w1314) -> ()  [unwired: 1 out]
                                n624 = call <userlib>:"Meadowlark USB Set Voltage.VI"("LC Voltage"=w1311, "LC Channel"=w1312, "FW Version"=w1313, "USB Open Device Cluster"=w1314) -> ()  [unwired: 1 out]
                                }
                                frame #1 {
                                n625 = Wait (ms)(milliseconds to wait=u32 35) -> ()  [unwired: 1 out]
                                }
                                }
                                }
                                frame #1 {
                                n626 = while {
                                shift-right: [w1326] -> w1320
                                shift-left: w1318 -> [w1329]
                                shift-right: [w1327] -> w1319
                                shift-left: w1317 -> [w1328]
                                stop <- w1325 continue-if-true
                                n627 = call <userlib>:"GetBusyStatus.vi"("error in (no error)"=w1328, "ph"=w1329) -> ("error out"=w1327:errorcluster, "BusyState"=w1325:bool, "hout"=w1326:u64)  [unwired: 2 in, 1 out]
                                }
                                n628 = while {
                                tunnel: w1320 -> [w1324]
                                shift-right: [w1321] -> w1316
                                shift-left: w1319 -> [w1322]
                                stop <- w1323 stop-if-true
                                n629 = call <userlib>:"ForceTrigger.vi"("ph"=w1324, "error in (no error)"=w1322) -> ("Triggered"=w1323:bool, "error out"=w1321:errorcluster)  [unwired: 1 in, 2 out]
                                }
                                }
                                frame #2 {
                                n630 = local read "Exposure in msec"() -> (w1331:u32)
                                n631 = Wait (ms)(milliseconds to wait=w1331) -> ()  [unwired: 1 out]
                                }
                                }
                                }
                                n632 = local read "Stop Spectroscopy sp"() -> (w1280:bool)
                              }
                            }
                            frame "Per Polarisation" {
                              n633 = for {
                                N: 4 -> [_]
                                tunnel: w1339 -> [w1347]
                                tunnel: w1337 -> [w1348]
                                shift-right: [w1346] -> w1340
                                shift-left: w1338 -> [w1345]
                                tunnel: w1335 -> [w1344]
                                tunnel: w1334 -> [w1343]
                                tunnel: w1333 -> [w1342]
                                tunnel: w1332 -> [w1341]
                                i -> [w1349]
                                n634 = flat-sequence {
                                tunnel: w1341 -> [w1353]
                                tunnel: w1342 -> [w1357]
                                tunnel: w1343 -> [w1358]
                                tunnel: w1344 -> [w1356]
                                tunnel: w1349 -> [w1359]
                                tunnel: w1348 -> [w1372]
                                tunnel: w1347 -> [w1371]
                                tunnel: [w1370] -> w1346
                                tunnel: w1345 -> [w1369]
                                frame #0 {
                                n635 = Index Array(array=w1357, index=w1359) -> (element=w1354:dbl)
                                n636 = Index Array(array=w1358, index=w1359) -> (element=w1351:dbl)
                                n637 = flat-sequence {
                                tunnel: [w1363] -> w1350
                                tunnel: w1354 -> [w1360]
                                tunnel: 2 ("LC Channel") -> [w1361]
                                tunnel: w1353 -> [w1362]
                                tunnel: w1356 -> [w1363]
                                tunnel: w1350 -> [w1367]
                                tunnel: w1353 -> [w1366]
                                tunnel: 1 ("LC Channel") -> [w1365]
                                tunnel: w1351 -> [w1364]
                                frame #0 {
                                n638 = call <userlib>:"Meadowlark USB Set Voltage.VI"("LC Voltage"=w1360, "LC Channel"=w1361, "FW Version"=w1362, "USB Open Device Cluster"=w1363) -> ()  [unwired: 1 out]
                                }
                                frame #1 {
                                n639 = call <userlib>:"Meadowlark USB Set Voltage.VI"("LC Voltage"=w1364, "LC Channel"=w1365, "FW Version"=w1366, "USB Open Device Cluster"=w1367) -> ()  [unwired: 1 out]
                                }
                                frame #2 {
                                n640 = Wait (ms)(milliseconds to wait=u32 35) -> ()  [unwired: 1 out]
                                }
                                }
                                }
                                frame #1 {
                                n641 = for {
                                N: w1372 -> [_]
                                tunnel: w1371 -> [w1379]
                                shift-right: [w1375] -> w1370
                                shift-left: w1369 -> [w1378]
                                stop <- w1374 stop-if-true
                                n642 = flat-sequence {
                                tunnel: w1379 -> [w1381]
                                tunnel: w1378 -> [w1380]
                                tunnel: [w1383] -> w1377
                                tunnel: [w1382] -> w1376
                                tunnel: w1377 -> [w1390]
                                tunnel: w1376 -> [w1389]
                                tunnel: [w1391] -> w1373
                                tunnel: [w1397] -> w1375
                                tunnel: w1373 -> [w1397]
                                frame #0 {
                                n643 = while {
                                shift-right: [w1386] -> w1382
                                shift-left: w1380 -> [w1387]
                                tunnel: w1381 -> [w1388]
                                tunnel: [w1385] -> w1383
                                stop <- w1384 continue-if-true
                                n644 = call <userlib>:"GetBusyStatus.vi"("error in (no error)"=w1387, "ph"=w1388) -> ("error out"=w1386:errorcluster, "BusyState"=w1384:bool, "hout"=w1385:u64)  [unwired: 2 in, 1 out]
                                }
                                }
                                frame #1 {
                                n645 = while {
                                tunnel: w1390 -> [w1395]
                                shift-right: [w1392] -> w1391
                                shift-left: w1389 -> [w1393]
                                stop <- w1394 stop-if-true
                                n646 = call <userlib>:"ForceTrigger.vi"("ph"=w1395, "error in (no error)"=w1393) -> ("Triggered"=w1394:bool, "error out"=w1392:errorcluster)  [unwired: 1 in, 2 out]
                                }
                                }
                                frame #2 {
                                n647 = local read "Exposure in msec"() -> (w1396:u32)
                                n648 = Wait (ms)(milliseconds to wait=w1396) -> ()  [unwired: 1 out]
                                }
                                }
                                n649 = local read "Stop Spectroscopy sp"() -> (w1374:bool)
                                }
                                }
                                }
                              }
                            }
                          }
                        }
                        frame #2 {
                          n650 = Get Date/Time In Seconds() -> (seconds since 1Jan1904=w1400:timestamp)
                          n651 = Build Array (concatenate)(w1398, w1400) -> (w1399:timestamp[])
                        }
                        frame #3 {
                          n652 = Wait (ms)(milliseconds to wait=w1404) -> ()  [unwired: 1 out]
                          n653 = call "helper_move_motor.vi"("Move step size"=w1401, "input cluster"=w1403) -> ("output cluster"=w1402:T14)  [unwired: 9 in]
                        }
                        frame #4 {
                          n654 = Wait (ms)(milliseconds to wait=u32 500) -> ()  [unwired: 1 out]
                        }
                      }
                      n655 = local write "Steps performed sp"(w1250) -> ()
                      n656 = local read "Scan distance (1=10nm) sp"() -> (w1246:dbl)
                      n657 = local read "Exposure in msec"() -> (w1249:u32)
                      n658 = local read "Motor Variable"() -> (w1248:T5)
                      n659 = local write "Motor Variable"(w1247) -> ()
                      n660 = local read "Stop Spectroscopy sp"() -> (w1252:bool)
                    }
                    "End time Array" <- w963
                    "Start time Array" <- w962
                  }
                  frame #4 {
                    n661 = Merge Errors(w1415, w1411) -> (w1414:errorcluster)
                    n662 = call <userlib>:"CancelImages.vi"("error in (no error)"=w1411, "ph"=w1412) -> ("error out"=w1408:errorcluster, "hout"=w1409:u64)  [unwired: 1 in, 1 out]
                    n663 = local read "Cam Variable"() -> (w1410:T6)
                    n664 = local read "Stop Spectroscopy sp"() -> (w1413:bool)
                    n665 = local read "spectroscopy/spectropolarimetry tab"() -> (w1406:enum32{"Spectroscopy", "Spectropolarimetry"})
                    n666 = call <vilib>:"Simple Error Handler.vi"("error in (no error)"=w1414) -> ()  [unwired: 4 in, 5 out]
                    n667 = Bundle(cluster=w1410, "hout"=w1409, "ErrorOut"=w1408) -> (w1407:T6)  [unwired: 1 in]
                    n668 = case shown="False" w1413 {
                      frame False {
                        n669 = Two Button Dialog(message="Spectropolarimetry completed successfully!!.    Reset Motor?", 1:"No" ("button name (\"OK\")"), 2:"Yes" ("T button name (\"OK\")")) -> (T button?=w1417:bool)
                        n670 = case shown="True" w1417 {
                          frame False {
                          }
                          frame True {
                            n671 = local read "Motor Variable"() -> (w1421:T5)
                            n672 = Unbundle By Name(w1421) -> ("Dup Controller #"=w1431:string, "VISA Refnum out"=w1430:refnum<visa-resource-name>, "DELAY (ms) out"=w1429:u32, "Move step size"=w1436:i32, "error out"=w1428:errorcluster)
                            n673 = call "get current and reset position.vi"("VISA Refnum in"=w1430, "DELAY (ms) in"=w1429, "Dup Controller # in"=w1431, "error in (no error)"=w1428) -> ("Dup Controller #"=w1427:string, "Reset displacement"=w1423:ext, "VISA Refnum out"=w1426:refnum<visa-resource-name>, "Delay (ms) out"=w1425:u32, "error out"=w1424:errorcluster)  [unwired: 9 in, 2 out]
                            n674 = while {
                              tunnel: [w1447] -> w1435
                              tunnel: [w1446] -> w1434
                              tunnel: [w1445] -> w1433
                              tunnel: [w1444] -> w1432
                              shift-right: [w1442] -> _
                              shift-left: w1423 -> [w1437]
                              tunnel: w1427 -> [w1441]
                              tunnel: w1426 -> [w1440]
                              tunnel: w1425 -> [w1439]
                              tunnel: w1424 -> [w1438]
                              stop <- w1443 stop-if-true
                              n675 = flat-sequence {
                                tunnel: [w1460] -> w1451
                                tunnel: [w1459] -> w1450
                                tunnel: [w1458] -> w1449
                                tunnel: [w1457] -> w1448
                                tunnel: w1441 -> [w1456]
                                tunnel: w1440 -> [w1455]
                                tunnel: w1439 -> [w1454]
                                tunnel: w1438 -> [w1453]
                                tunnel: w1437 -> [w1452]
                                tunnel: w1451 -> [w1472]
                                tunnel: w1450 -> [w1471]
                                tunnel: w1449 -> [w1469]
                                tunnel: w1448 -> [w1470]
                                tunnel: [w1468] -> w1447
                                tunnel: [w1467] -> w1446
                                tunnel: [w1466] -> w1445
                                tunnel: [w1465] -> w1444
                                tunnel: [w1463] -> w1443
                                tunnel: [w1462] -> w1442
                                frame #0 {
                                n676 = call "motor motion and reset.vi"("VISA Refnum in"=w1455, "Dup Controller # in"=w1456, "DELAY (ms) in"=w1454, "Reset"=TRUE, "error in (no error)"=w1453, "Reset displacement"=w1452) -> ("DELAY (ms) out"=w1458:u32, "VISA Refnum out"=w1459:refnum<visa-resource-name>, "Dup Controller # out"=w1460:string, "error out"=w1457:errorcluster)  [unwired: 4 in, 2 out]
                                }
                                frame #1 {
                                n677 = call "get current and reset position.vi"("VISA Refnum in"=w1471, "DELAY (ms) in"=w1469, "Dup Controller # in"=w1472, "error in (no error)"=w1470) -> ("Dup Controller #"=w1468:string, "Reset displacement"=w1462:ext, "VISA Refnum out"=w1466:refnum<visa-resource-name>, "Delay (ms) out"=w1467:u32, "Current position"=w1464:i32, "error out"=w1465:errorcluster)  [unwired: 9 in, 1 out]
                                n678 = Equal To 0?(x=w1464) -> (x = 0?=w1463:bool)
                                }
                              }
                            }
                            n679 = Bundle("Dup Controller #"=w1435, "VISA Refnum out"=w1433, "Delay (ms) out"=w1434, "Move step size"=w1436, "error out"=w1432) -> (w1422:T15)  [unwired: 1 in]
                            n680 = local write "Motor Variable"(w1422) -> ()
                          }
                        }
                      }
                      frame True {
                        n681 = local write "Stop Spectroscopy sp"(FALSE ("Stop Spectroscopy sp")) -> ()
                        n682 = Two Button Dialog(message="Spectroscopy Stopped by user. Reset motor?", 1:"No" ("F button name (\"Cancel\")"), 2:"Yes" ("T button name (\"OK\")")) -> (T button?=w1474:bool)
                        n683 = case shown="True" w1474 {
                          frame False {
                          }
                          frame True {
                            n684 = local read "Motor Variable"() -> (w1479:T5)
                            n685 = Unbundle By Name(w1479) -> ("Dup Controller #"=w1488:string, "VISA Refnum out"=w1487:refnum<visa-resource-name>, "DELAY (ms) out"=w1486:u32, "Move step size"=w1493:i32, "error out"=w1485:errorcluster)
                            n686 = call "get current and reset position.vi"("VISA Refnum in"=w1487, "DELAY (ms) in"=w1486, "Dup Controller # in"=w1488, "error in (no error)"=w1485) -> ("Dup Controller #"=w1484:string, "Reset displacement"=w1480:ext, "VISA Refnum out"=w1483:refnum<visa-resource-name>, "Delay (ms) out"=w1482:u32, "error out"=w1481:errorcluster)  [unwired: 9 in, 2 out]
                            n687 = while {
                              tunnel: [w1504] -> w1492
                              tunnel: [w1503] -> w1491
                              tunnel: [w1502] -> w1490
                              tunnel: [w1501] -> w1489
                              shift-right: [w1499] -> _
                              shift-left: w1480 -> [w1494]
                              tunnel: w1484 -> [w1498]
                              tunnel: w1483 -> [w1497]
                              tunnel: w1482 -> [w1496]
                              tunnel: w1481 -> [w1495]
                              stop <- w1500 stop-if-true
                              n688 = flat-sequence {
                                tunnel: [w1517] -> w1508
                                tunnel: [w1516] -> w1507
                                tunnel: [w1515] -> w1506
                                tunnel: [w1514] -> w1505
                                tunnel: w1498 -> [w1513]
                                tunnel: w1497 -> [w1512]
                                tunnel: w1496 -> [w1511]
                                tunnel: w1495 -> [w1510]
                                tunnel: w1494 -> [w1509]
                                tunnel: w1508 -> [w1529]
                                tunnel: w1507 -> [w1528]
                                tunnel: w1506 -> [w1526]
                                tunnel: w1505 -> [w1527]
                                tunnel: [w1525] -> w1504
                                tunnel: [w1524] -> w1503
                                tunnel: [w1523] -> w1502
                                tunnel: [w1522] -> w1501
                                tunnel: [w1520] -> w1500
                                tunnel: [w1519] -> w1499
                                frame #0 {
                                n689 = call "motor motion and reset.vi"("VISA Refnum in"=w1512, "Dup Controller # in"=w1513, "DELAY (ms) in"=w1511, "Reset"=TRUE, "error in (no error)"=w1510, "Reset displacement"=w1509) -> ("DELAY (ms) out"=w1515:u32, "VISA Refnum out"=w1516:refnum<visa-resource-name>, "Dup Controller # out"=w1517:string, "error out"=w1514:errorcluster)  [unwired: 4 in, 2 out]
                                }
                                frame #1 {
                                n690 = call "get current and reset position.vi"("VISA Refnum in"=w1528, "DELAY (ms) in"=w1526, "Dup Controller # in"=w1529, "error in (no error)"=w1527) -> ("Dup Controller #"=w1525:string, "Reset displacement"=w1519:ext, "VISA Refnum out"=w1523:refnum<visa-resource-name>, "Delay (ms) out"=w1524:u32, "Current position"=w1521:i32, "error out"=w1522:errorcluster)  [unwired: 9 in, 1 out]
                                n691 = Equal To 0?(x=w1521) -> (x = 0?=w1520:bool)
                                }
                              }
                            }
                            n692 = Bundle("Dup Controller #"=w1492, "VISA Refnum out"=w1490, "Delay (ms) out"=w1491, "Move step size"=w1493, "error out"=w1489) -> (w1478:T15)  [unwired: 1 in]
                            n693 = local write "Motor Variable"(w1478) -> ()
                          }
                        }
                      }
                    }
                    n694 = local write "Cam Variable"(w1407) -> ()
                    n695 = case shown="\"Spectropolarimetry\"" w1406 {
                      frame "Spectroscopy" {
                      }
                      frame "Spectropolarimetry" {
                        n696 = local read "LCVR closing\nvariable"() -> (w1416:T1)
                        n697 = call "Meadowlark USB Easy Close.vi"("USB Device and Pipes Array"=w1416) -> ()
                      }
                    }
                  }
                }
                n698 = local read "LCVR variable"() -> (w722:T2)
                n699 = Unbundle By Name(w722) -> ("Open USB I/O Stuff"=w723:T10, "Current Lcvr Temp"=w724:dbl)  [unwired: 1 out]
                n700 = while {
                  shift-right: [w741] -> w721
                  shift-left: w723 -> [w741]
                  shift-right: [w746] -> w719
                  shift-left: w724 -> [w740]
                  i -> [w734]
                  stop <- w736 stop-if-true
                  n701 = call "read temp.vi"("USB Open Device Cluster"=w741) -> ("Temp"=w746:dbl)
                  n702 = local read "Stop Spectroscopy sp"() -> (w737:bool)
                  n703 = Equal?(x=w734, y=10) -> (x = y?=w732:bool)
                  n704 = local read "Close USO software"() -> (w738:bool)
                  n705 = local read "LCVR Temperature in deg C\n      Set         Current"() -> (w745:dbl[])
                  n706 = Compound Arithmetic op=OR(w738, w737, w732) -> (w736:bool)
                  n707 = local read "LCVR Set Temperature"() -> (w742:dbl)
                  n708 = Index Array(array=w745, index=0) -> (element=w735:dbl)
                  n709 = Not Equal?(x=w735, y=w742) -> (x != y?=w743:bool)
                  n710 = Build Array(w735, w740) -> (w739:dbl[])
                  n711 = case shown="True" w743 {
                    tunnel: w735 -> [_ w747]
                    tunnel: w741 -> [_ w748]
                    frame False {
                    }
                    frame True {
                      n712 = call "Set temp.vi"("Temp"=w747, "USB Open Device Cluster"=w748) -> ()  [unwired: 1 in]
                      n713 = local write "LCVR Set Temperature"(w747) -> ()
                    }
                  }
                  n714 = local write "LCVR Temperature in deg C\n      Set         Current"(w739) -> ()
                }
                n715 = Bundle By Name(cluster=w722, "Open USB I/O Stuff"=w721, "Current Lcvr Temp"=w719) -> (w720:T2)
                n716 = local write "LCVR variable"(w720) -> ()
              }
            }
          }
          frame True {
          }
        }
        n717 = Or(x="Close USO software", y=w262) -> (x .or. y?=w263:bool)
      }
      n718 = property on="Scan distance (1=10nm)" class="DigNum (strict)"("Value"=w259) -> ()  [unwired: 2 in, 2 out]
      n719 = property on="Scan distance (1=10nm) sp" class="DigNum (strict)"("Value"=w259) -> ()  [unwired: 2 in, 2 out]
      n720 = Build Array(w257, w256) -> (w255:dbl[])
      n721 = property on="LCVR Temperature in deg C\n      Set         Current" class="Arr (strict)"("Value"=w255) -> ()  [unwired: 2 in, 2 out]
    }
  }
  n722 = property on="CCD Display" class="IntGraph (strict)"("XScale.Minimum"=w4) -> ()  [unwired: 2 in, 2 out]
  n723 = property on="CCD Display" class="IntGraph (strict)"("YScale.Minimum"=w4) -> ()  [unwired: 2 in, 2 out]
  n724 = property on="Finish" class="Bool"("Visible"=w1) -> ()  [unwired: 2 in, 2 out]
  n725 = property on="Slide" class="Slide (strict)"("Visible"=w1) -> ()  [unwired: 2 in, 2 out]
  n726 = property on="Slide sp" class="Slide (strict)"("Visible"=w1) -> ()  [unwired: 2 in, 2 out]
  n727 = property on="Status" class="Str"("Visible"=w1) -> ()  [unwired: 2 in, 2 out]
  n728 = property on="Apply" class="Bool (strict)"("Visible"=w1) -> ()  [unwired: 2 in, 2 out]
  n729 = property on="CCD Display" class="IntGraph (strict)"("YScale.Maximum"=w3) -> ()  [unwired: 2 in, 2 out]
  n730 = property on="CCD Display" class="IntGraph (strict)"("XScale.Maximum"=w3) -> ()  [unwired: 2 in, 2 out]
  n731 = property on="Voltage-Retardance file path for lcvr2" class="Path"("Visible"=w1) -> ()  [unwired: 2 in, 2 out]
  n732 = property on="Move step size(1=10nm)" class="DigNum (strict)"("Visible"=w1) -> ()  [unwired: 2 in, 2 out]
  n733 = property on="VISA Refnum in" class="VISAName"("Visible"=w1) -> ()  [unwired: 2 in, 2 out]
  n734 = property on="CONTROLLER Number" class="Str"("Visible"=w1) -> ()  [unwired: 2 in, 2 out]
  n735 = property on="DELAY (ms) in" class="DigNum (strict)"("Visible"=w1) -> ()  [unwired: 2 in, 2 out]
  n736 = property on="Initialise Device" class="Ring (strict)"("Visible"=w1) -> ()  [unwired: 2 in, 2 out]
  n737 = property on="Close USO software" class="Bool (strict)"("Visible"=w1) -> ()  [unwired: 2 in, 2 out]
  n738 = property on="accept intensity" class="Bool (strict)"("Visible"=w1) -> ()  [unwired: 2 in, 2 out]
  n739 = property on="LCVR Set Temperature" class="DigNum (strict)"("Visible"=w1) -> ()  [unwired: 2 in, 2 out]
  n740 = property on="Voltage-Retardance file path for lcvr1" class="Path"("Visible"=w1) -> ()  [unwired: 2 in, 2 out]
  n741 = property on="accept intensity sp" class="Bool (strict)"("Visible"=w1) -> ()  [unwired: 2 in, 2 out]
  n742 = property on="Start observation session" class="Bool (strict)"("Visible"=w1) -> ()  [unwired: 2 in, 2 out]
  n743 = property on="Delay in msec" class="DigNum (strict)"("Visible"=w1) -> ()  [unwired: 2 in, 2 out]
  n744 = property on="Exposure in msec" class="DigNum (strict)"("Visible"=w1) -> ()  [unwired: 2 in, 2 out]
  n745 = property on="InterfaceType" class="Ring (strict)"("Visible"=w1) -> ()  [unwired: 2 in, 2 out]
  n746 = property on="spectroscopy/spectropolarimetry tab" class="TabCtl (strict)"("Visible"=w1) -> ()  [unwired: 2 in, 2 out]
  "Buf no 2" <- w2
  "Buf no 1" <- w2
